vi "recorder.vi"() -> ()   [LabVIEW 2022 SP3]
uses:
  <vilib>/DAQmx/write.llb/DAQmx Write (Digital 1D Bool 1Chan 1Samp).vi
  <vilib>/Utility/file.llb/Write Delimited Spreadsheet (DBL).vi
  <vilib>/Utility/inputDevices.llb/keyboardAcquire.vi
  <vilib>/DAQmx/create/channels.llb/DAQmx Create Channel (DO-Digital Output).vi
  <vilib>/DAQmx/miscellaneous.llb/DAQmx Fill In Error Info.vi
panel:
  out "Array":dbl[](array[numeric])
  out "Numeric":dbl
  out "error out 97":errorcluster
  out "error out 96":errorcluster
  out "error out 95":errorcluster
  out "error out 94":errorcluster
  out "error out 93":errorcluster
  out "error out 92":errorcluster
  out "error out 91":errorcluster
  out "error out 90":errorcluster
  out "error out 89":errorcluster
  out "error out 88":errorcluster
  out "error out 87":errorcluster
  out "error out 86":errorcluster
  out "error out 85":errorcluster
  out "error out 84":errorcluster
  out "error out 83":errorcluster
  out "error out 82":errorcluster
  out "error out 81":errorcluster
  out "error out 80":errorcluster
  out "error out 79":errorcluster
  out "error out 78":errorcluster
  out "error out 77":errorcluster
  out "error out 76":errorcluster
  out "error out 75":errorcluster
  out "error out 74":errorcluster
  out "error out 73":errorcluster
  out "error out 72":errorcluster
  out "error out 71":errorcluster
  out "error out 70":errorcluster
  out "error out 69":errorcluster
  out "error out 68":errorcluster
  out "error out 67":errorcluster
  out "error out 66":errorcluster
  out "error out 65":errorcluster
  out "error out 64":errorcluster
  out "error out 63":errorcluster
  out "error out 62":errorcluster
  out "error out 61":errorcluster
  out "error out 60":errorcluster
  out "error out 59":errorcluster
  out "error out 58":errorcluster
  out "error out 57":errorcluster
  out "error out 56":errorcluster
  out "error out 55":errorcluster
  out "error out 54":errorcluster
  out "error out 53":errorcluster
  out "error out 52":errorcluster
  out "error out 51":errorcluster
  out "error out 50":errorcluster
  out "error out 49":errorcluster
  out "error out 48":errorcluster
  out "error out 47":errorcluster
  out "error out 46":errorcluster
  out "error out 45":errorcluster
  out "error out 44":errorcluster
  out "error out 43":errorcluster
  out "error out 42":errorcluster
  out "error out 41":errorcluster
  out "error out 40":errorcluster
  out "error out 39":errorcluster
  out "error out 38":errorcluster
  out "error out 37":errorcluster
  out "error out 36":errorcluster
  out "error out 35":errorcluster
  out "error out 34":errorcluster
  out "error out 33":errorcluster
  out "error out 32":errorcluster
  out "error out 31":errorcluster
  out "error out 30":errorcluster
  out "error out 29":errorcluster
  out "error out 28":errorcluster
  out "error out 27":errorcluster
  out "error out 26":errorcluster
  out "error out 18":errorcluster
  out "error out 19":errorcluster
  out "error out 20":errorcluster
  out "error out 21":errorcluster
  out "error out 22":errorcluster
  out "error out 23":errorcluster
  out "error out 24":errorcluster
  out "error out 25":errorcluster
  in  "stop":bool
  out "key":T1(ring)
  out "String":string
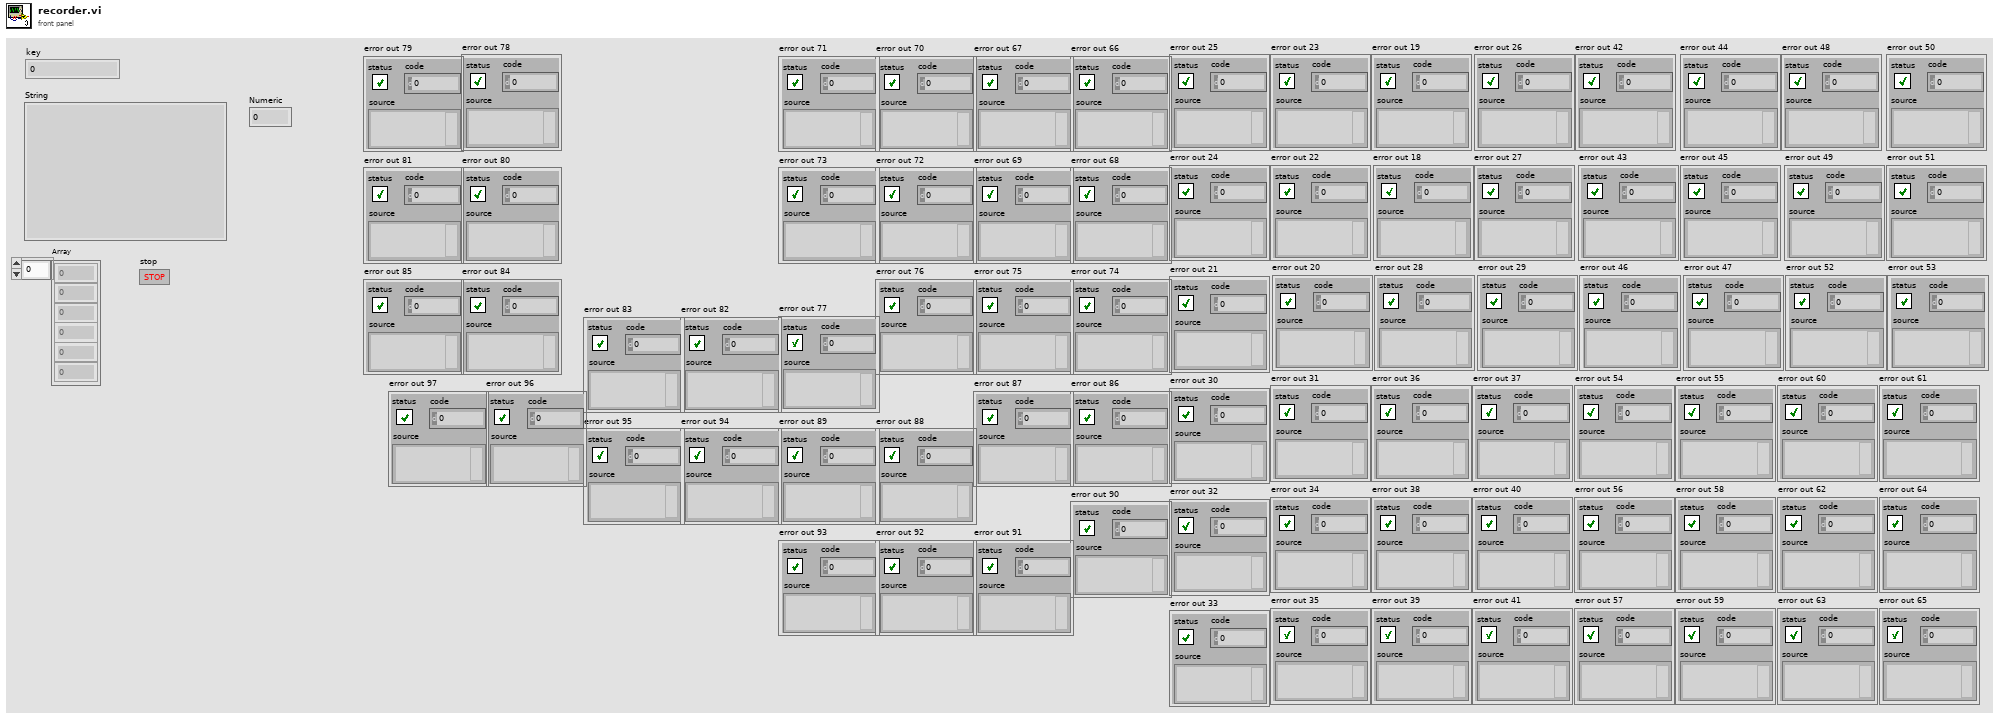
[diagram p1: front panel]
types:
  T1 = enum16{"0", "1", "2", "3", "4", "5", "6", "7", "8", "9", "A", "B", "C", "D", "E", "F", "G", "H", "I", "J", "K", "L", "M", "N", "O", "P", "Q", "R", "S", "T", "U", "V", "W", "X", "Y", "Z", "F1", "F2", "F3", "F4", "F5", "F6", "F7", "F8", "F9", "F10", "F11", "F12", "F13", "F14", "F15", "ADD", "BACK", "BACKSLASH", "CAPITAL", "COMMA", "DECIMAL", "DELETE", "DIVIDE", "DOWN", "END", "EQUALS", "ESCAPE", "GRAVE (`)", "HOME", "INSERT", "LBRACKET", "LCONTROL", "LEFT", "L ALT", "LSHIFT", "LWIN", "MINUS", "MULTIPLY", "NEXT", "NUMLOCK", "NUMPAD_0", "NUMPAD_1", "NUMPAD_2", "NUMPAD_3", "NUMPAD_4", "NUMPAD_5", "NUMPAD_6", "NUMPAD_7", "NUMPAD_8", "NUMPAD_9", "PAUSE", "PERIOD", "PRIOR (PG UP)", "RBRACKET", "RCONTROL", "RETURN", "RIGHT", "R ALT", "RSHIFT", "RWIN", "SCROLL", "SEMICOLON", "SLASH", "SPACE", "SUBTRACT", "TAB", "UP", "ENTER (num pad)", "' (quote)"}
  T2 = enum16{"0", "1", "2", "3", "4", "5", "6", "7", "8", "9", "A", "B", "C", "D", "E", "F", "G", "H", "I", "J", "K", "L", "M", "N", "O", "P", "Q", "R", "S", "T", "U", "V", "W", "X", "Y", "Z", "F1", "F2", "F3", "F4", "F5", "F6", "F7", "F8", "F9", "F10", "F11", "F12", "F13", "F14", "F15", "ADD", "BACK", "BACKSLASH", "CAPITAL", "COMMA", "DECIMAL", "DELETE", "DIVIDE", "DOWN", "END", "EQUALS", "ESCAPE", "GRAVE (`)", "HOME", "INSERT", "LBRACKET", "LCONTROL", "LEFT", "L ALT", "LSHIFT", "LWIN", "MINUS", "MULTIPLY", "NEXT", "NUMLOCK", "NUMPAD_0", "NUMPAD_1", "NUMPAD_2", "NUMPAD_3", "NUMPAD_4", "NUMPAD_5", "NUMPAD_6", "NUMPAD_7", "NUMPAD_8", "NUMPAD_9", "PAUSE", "PERIOD", "PRIOR (PG UP)", "RBRACKET", "RCONTROL", "RETURN", "RIGHT", "R ALT", "RSHIFT", "RWIN", "SCROLL", "SEMICOLON", "SLASH", "SPACE", "SUBTRACT", "TAB", "UP", "ENTER (num pad)", "' (quote)"}[]
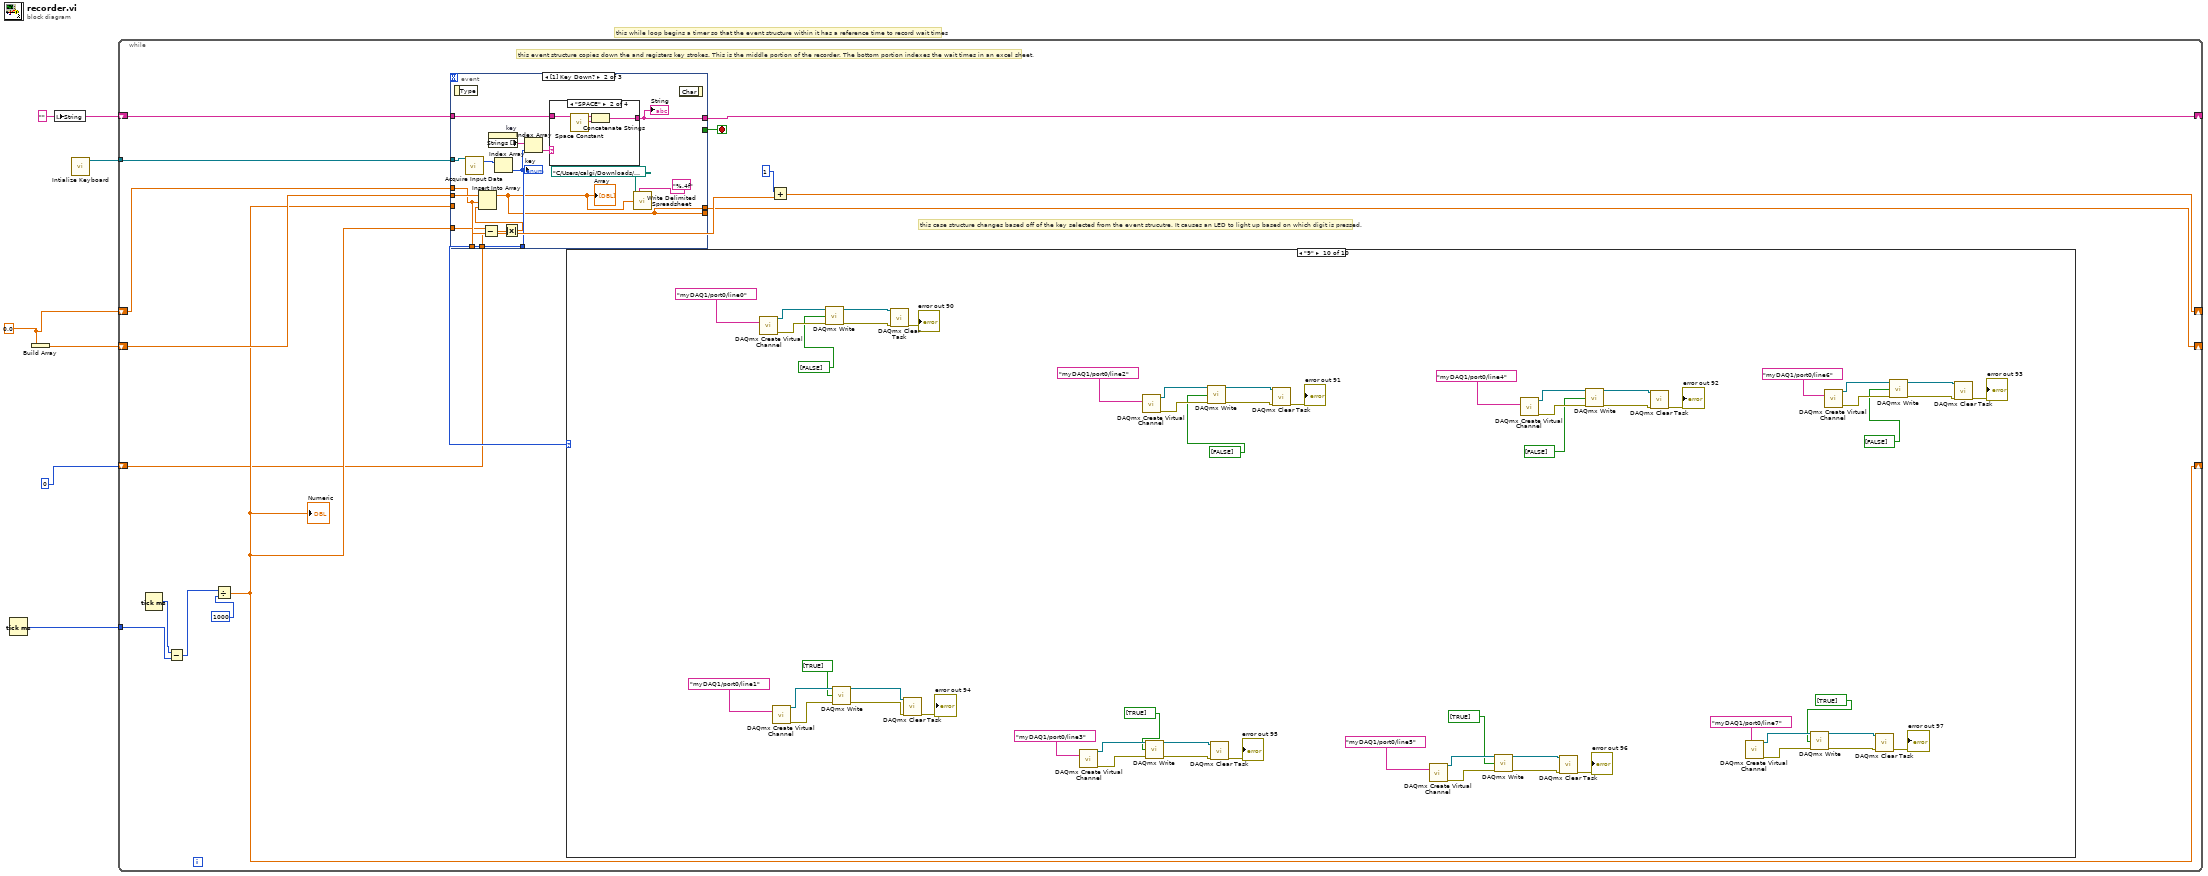
[diagram p0: block diagram]
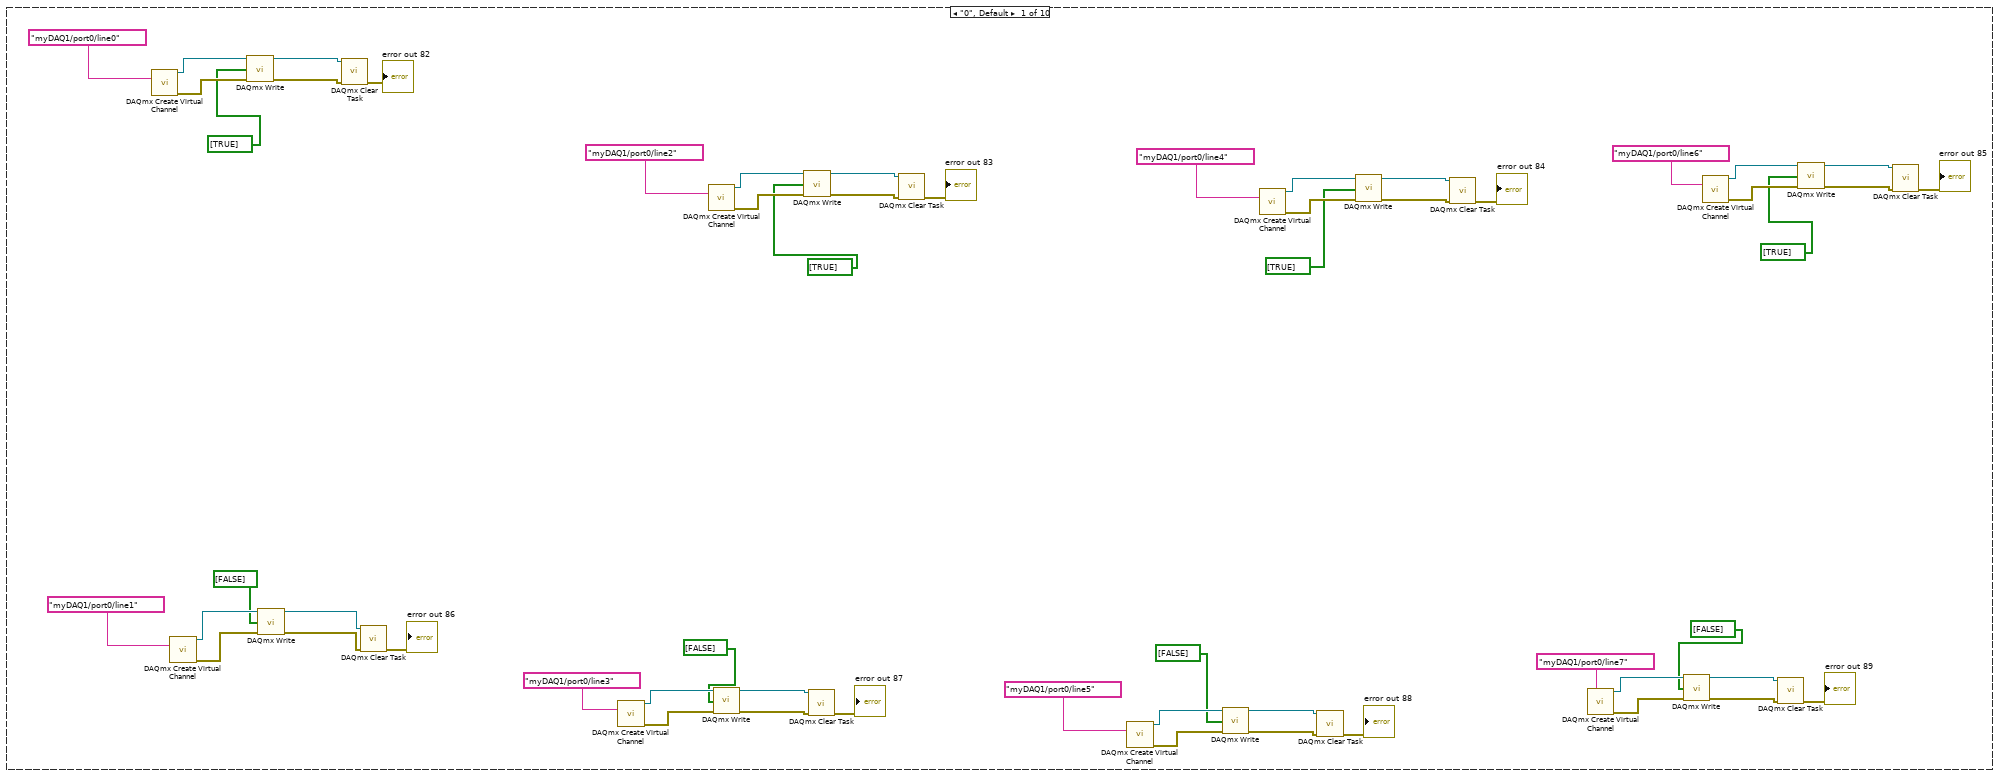
[diagram p2: hidden frame]
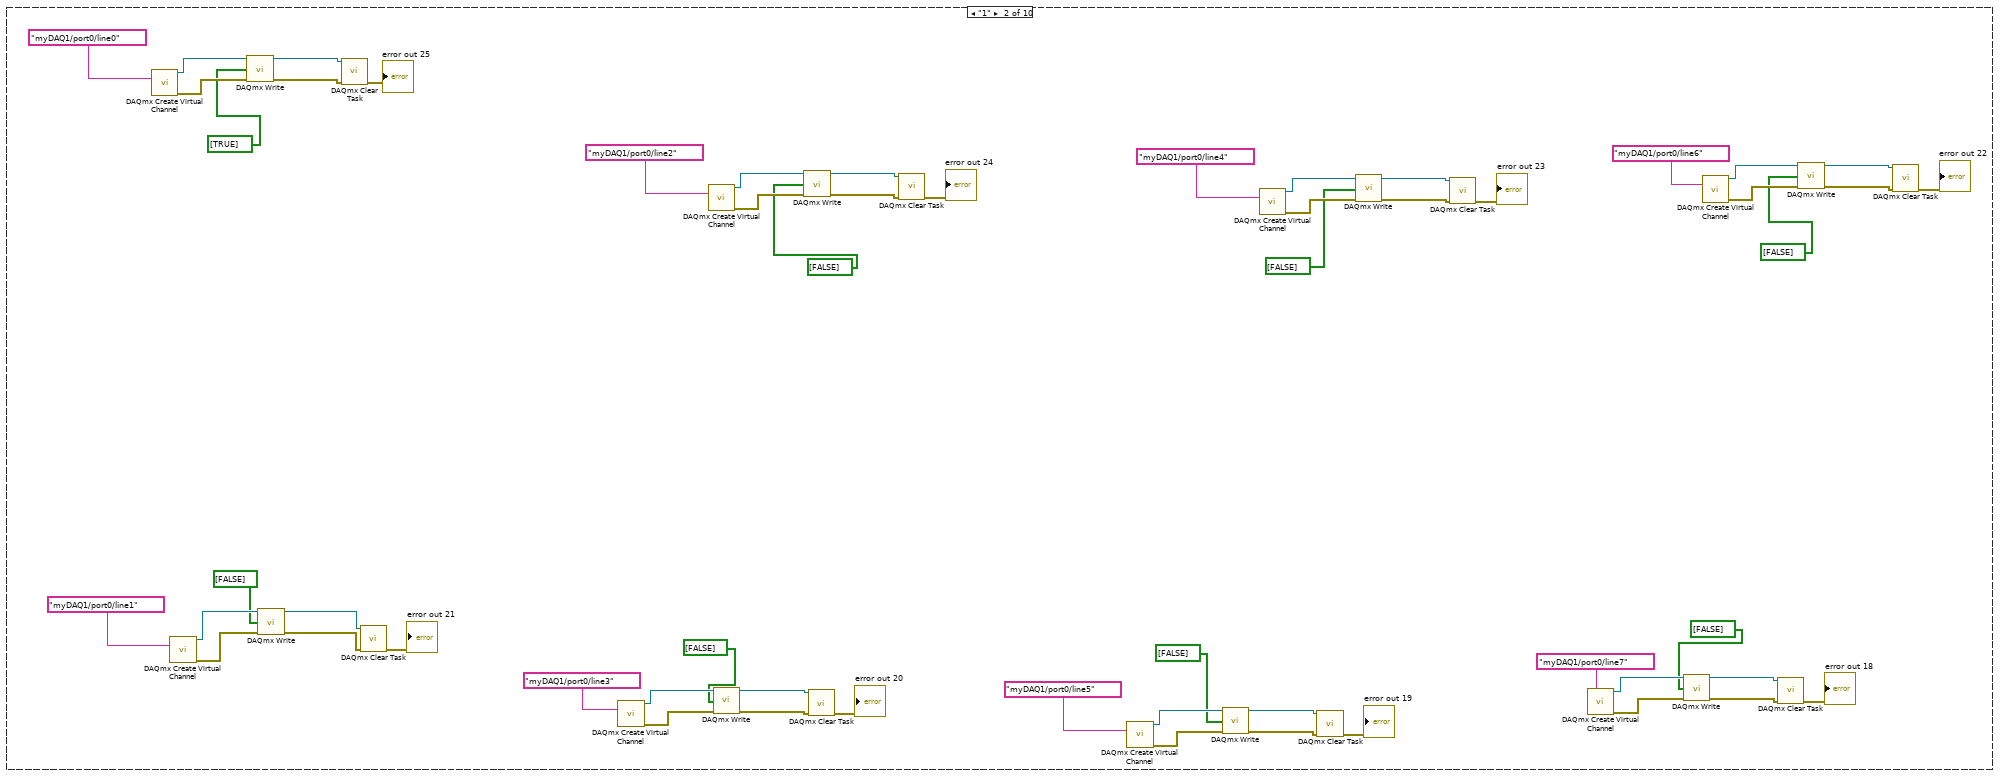
[diagram p3: hidden frame]
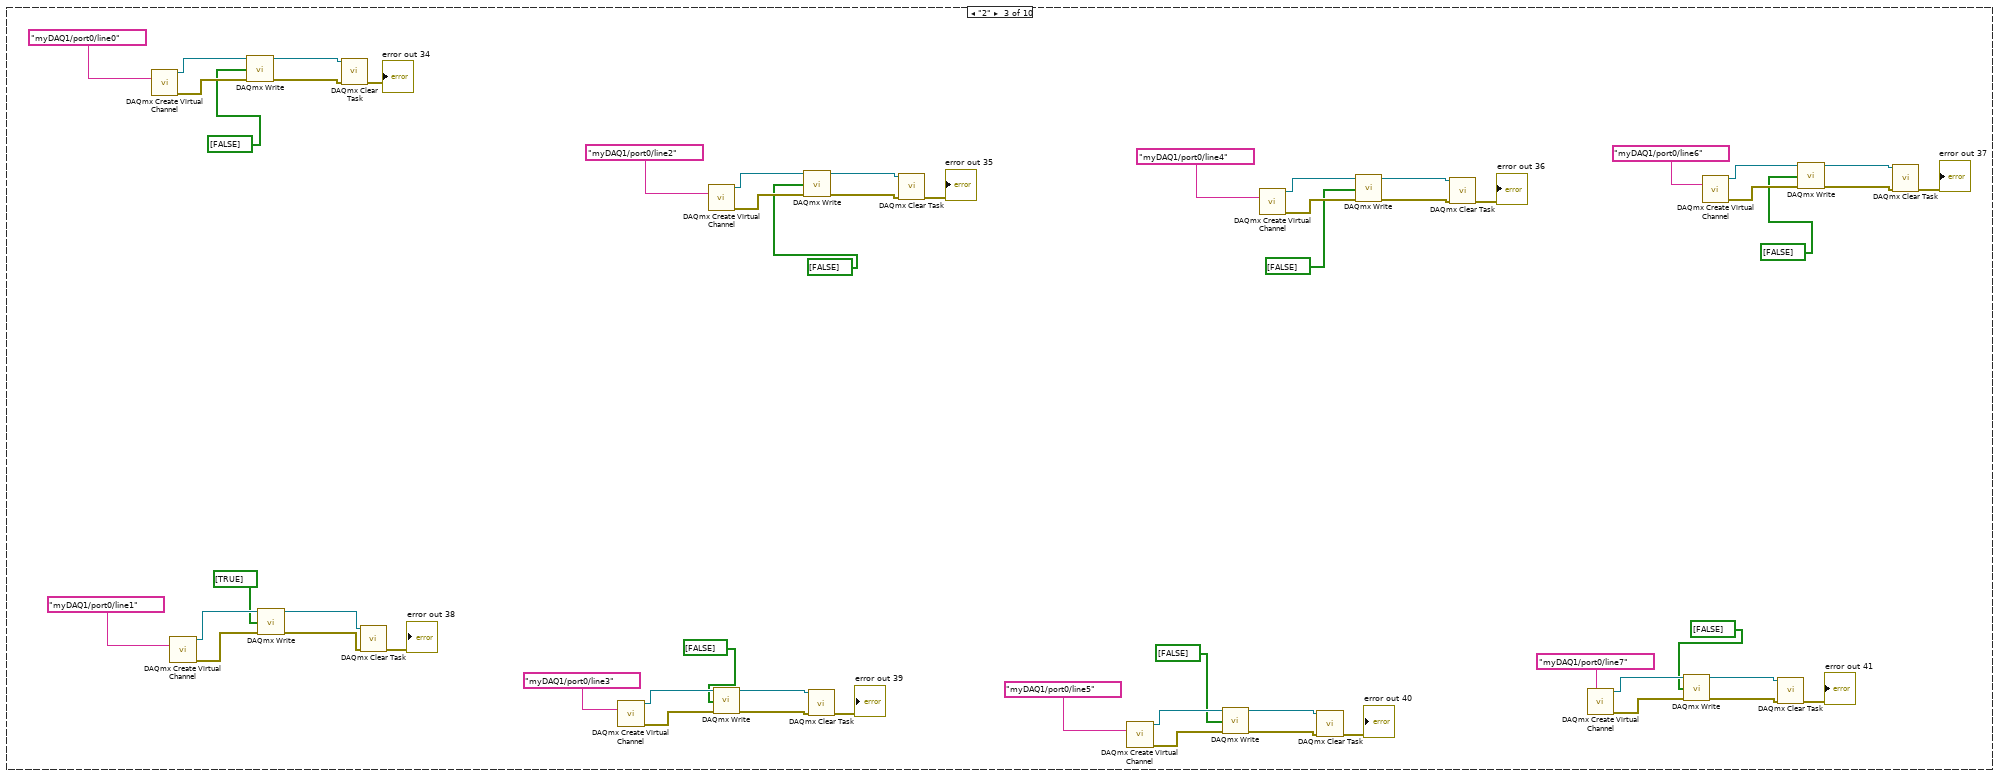
[diagram p4: hidden frame]
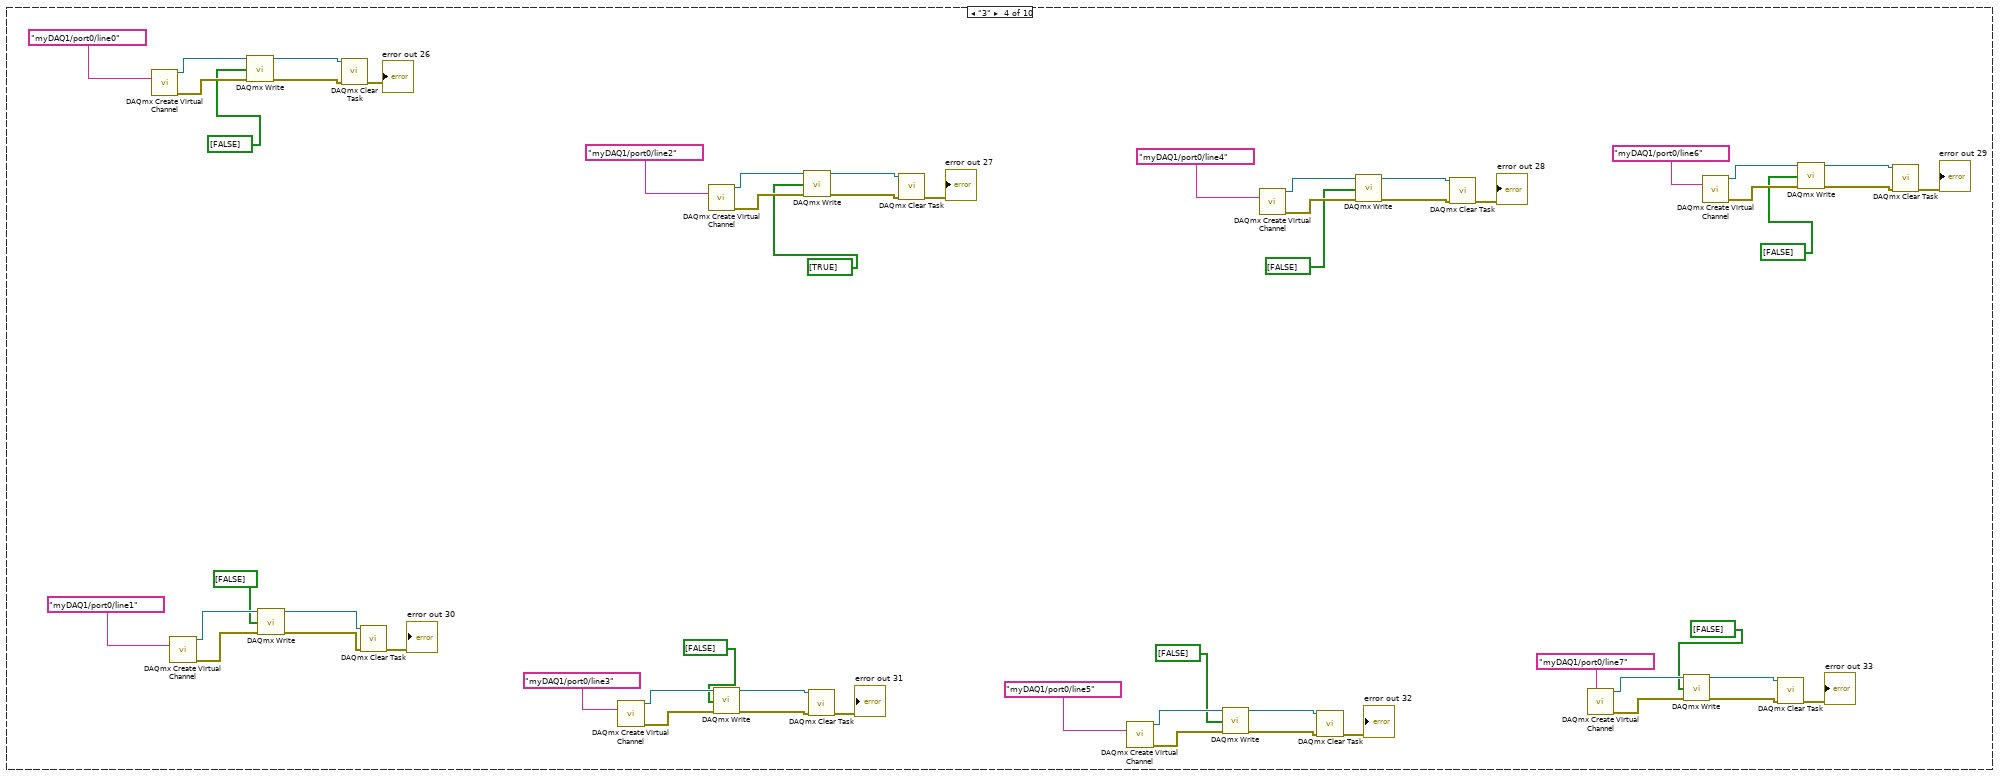
[diagram p5: hidden frame]
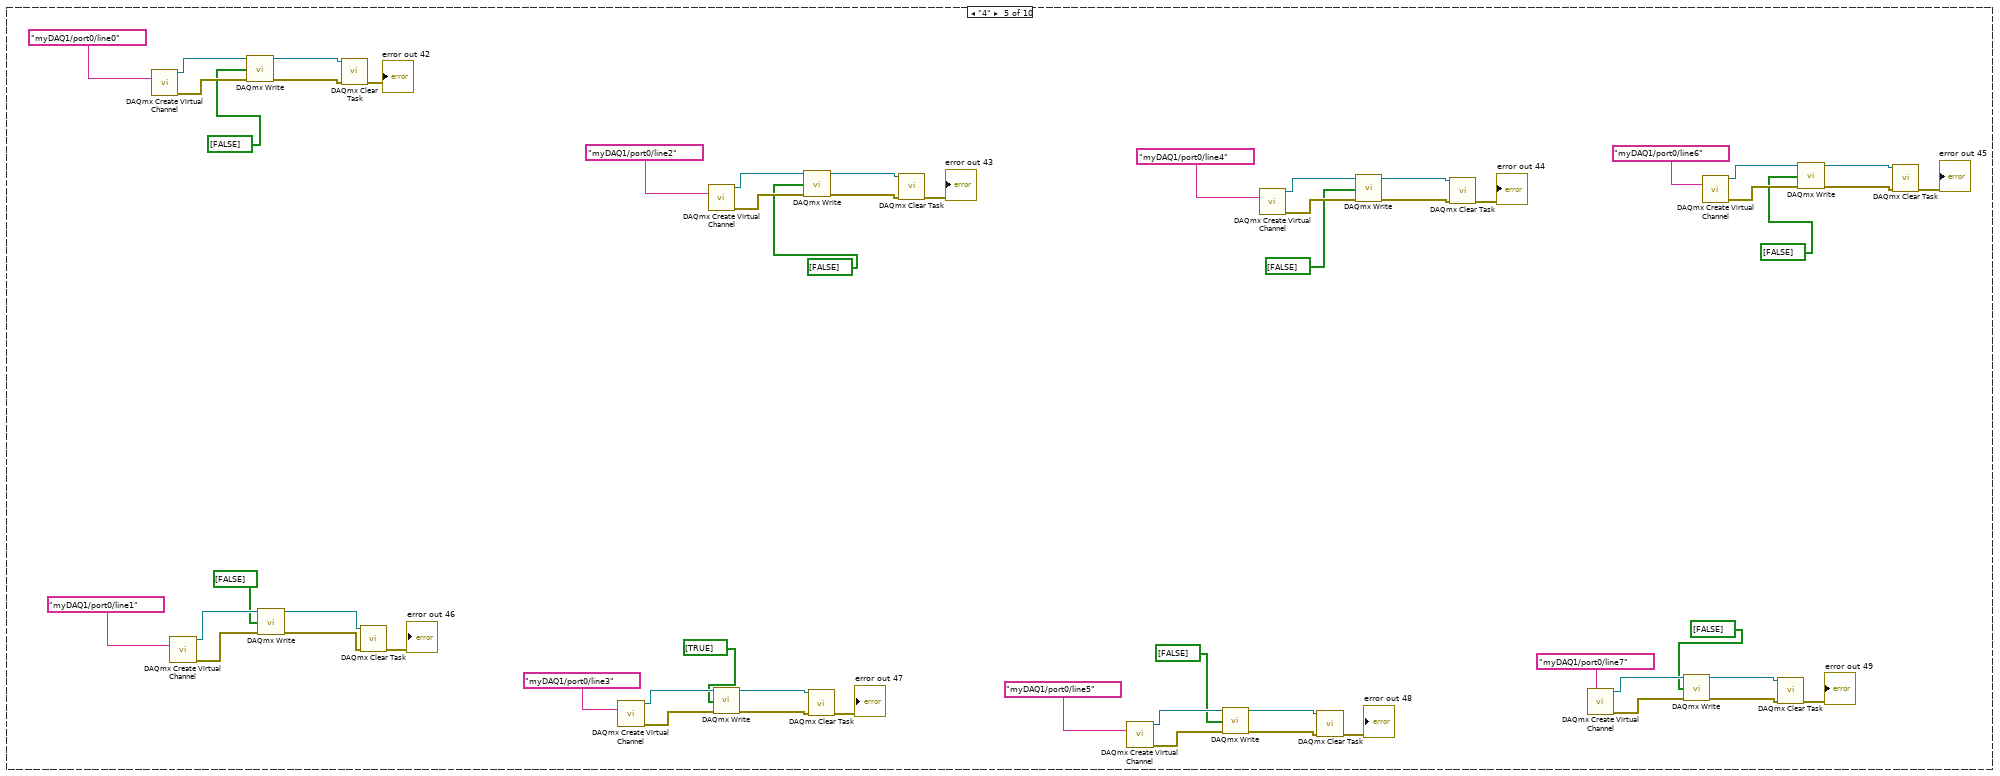
[diagram p6: hidden frame]
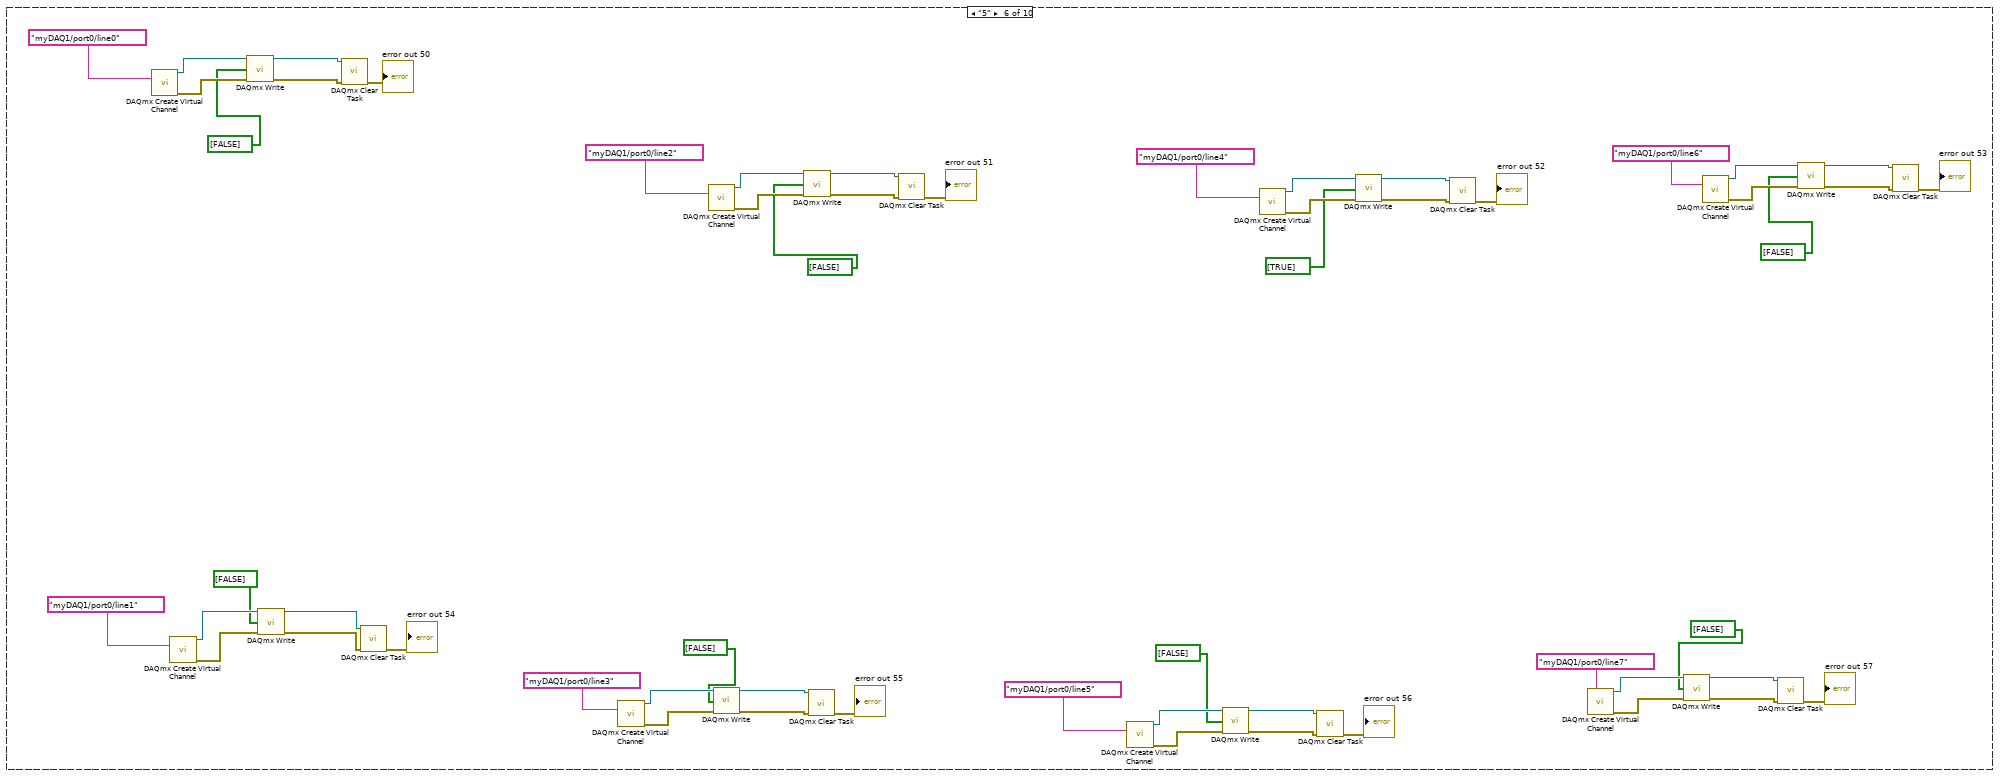
[diagram p7: hidden frame]
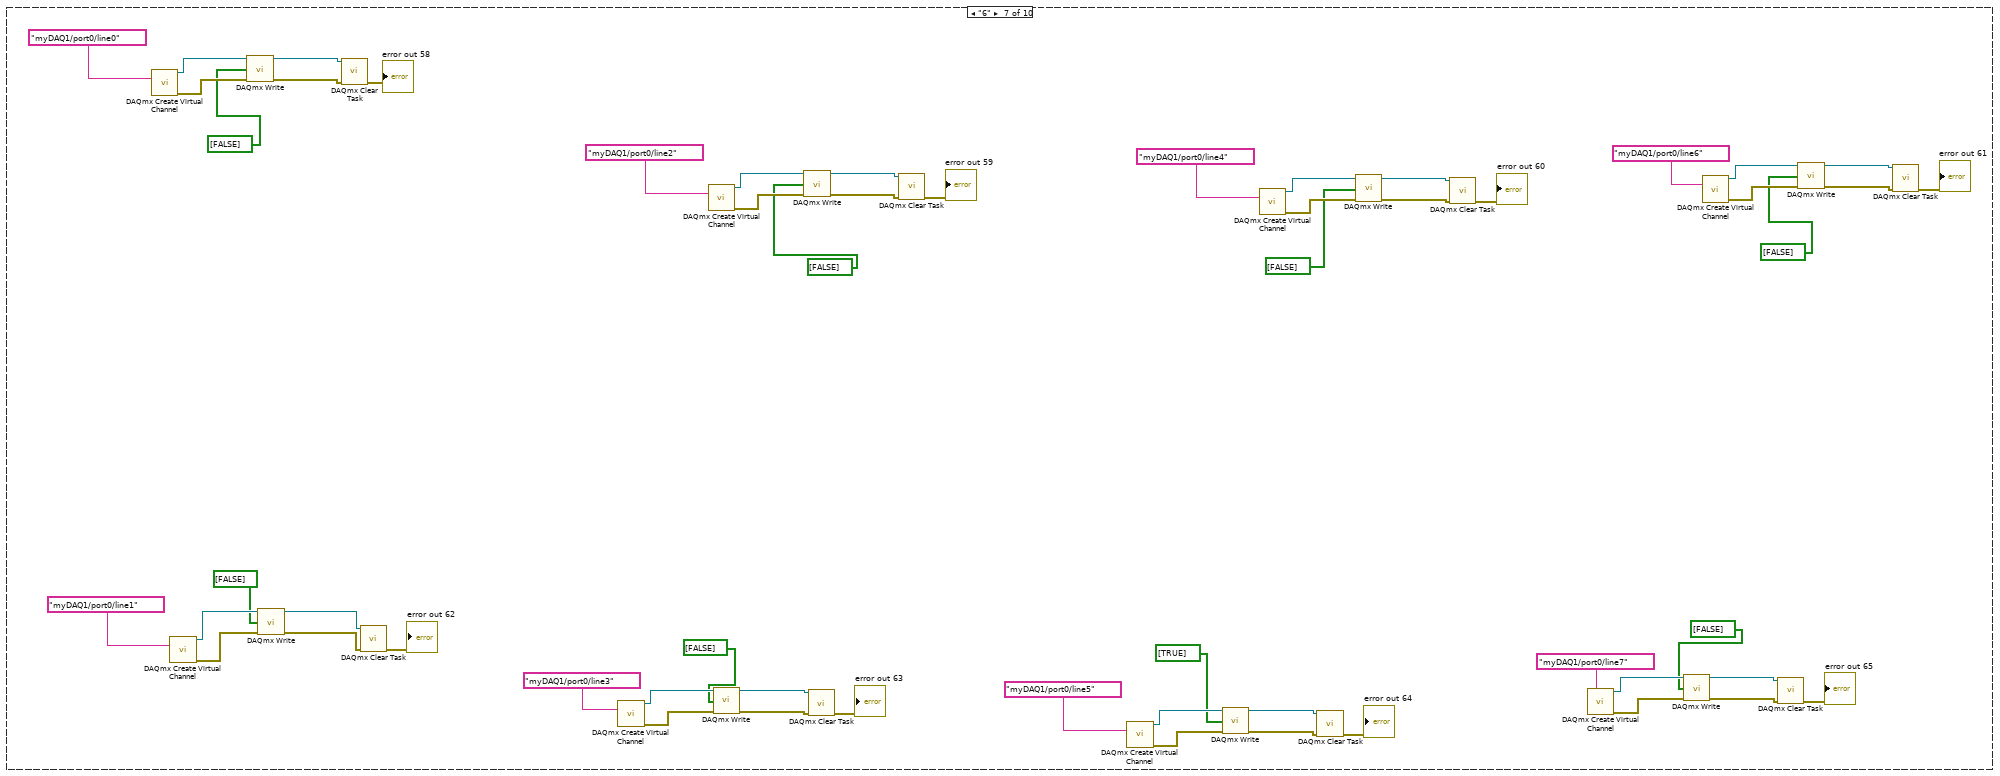
[diagram p8: hidden frame]
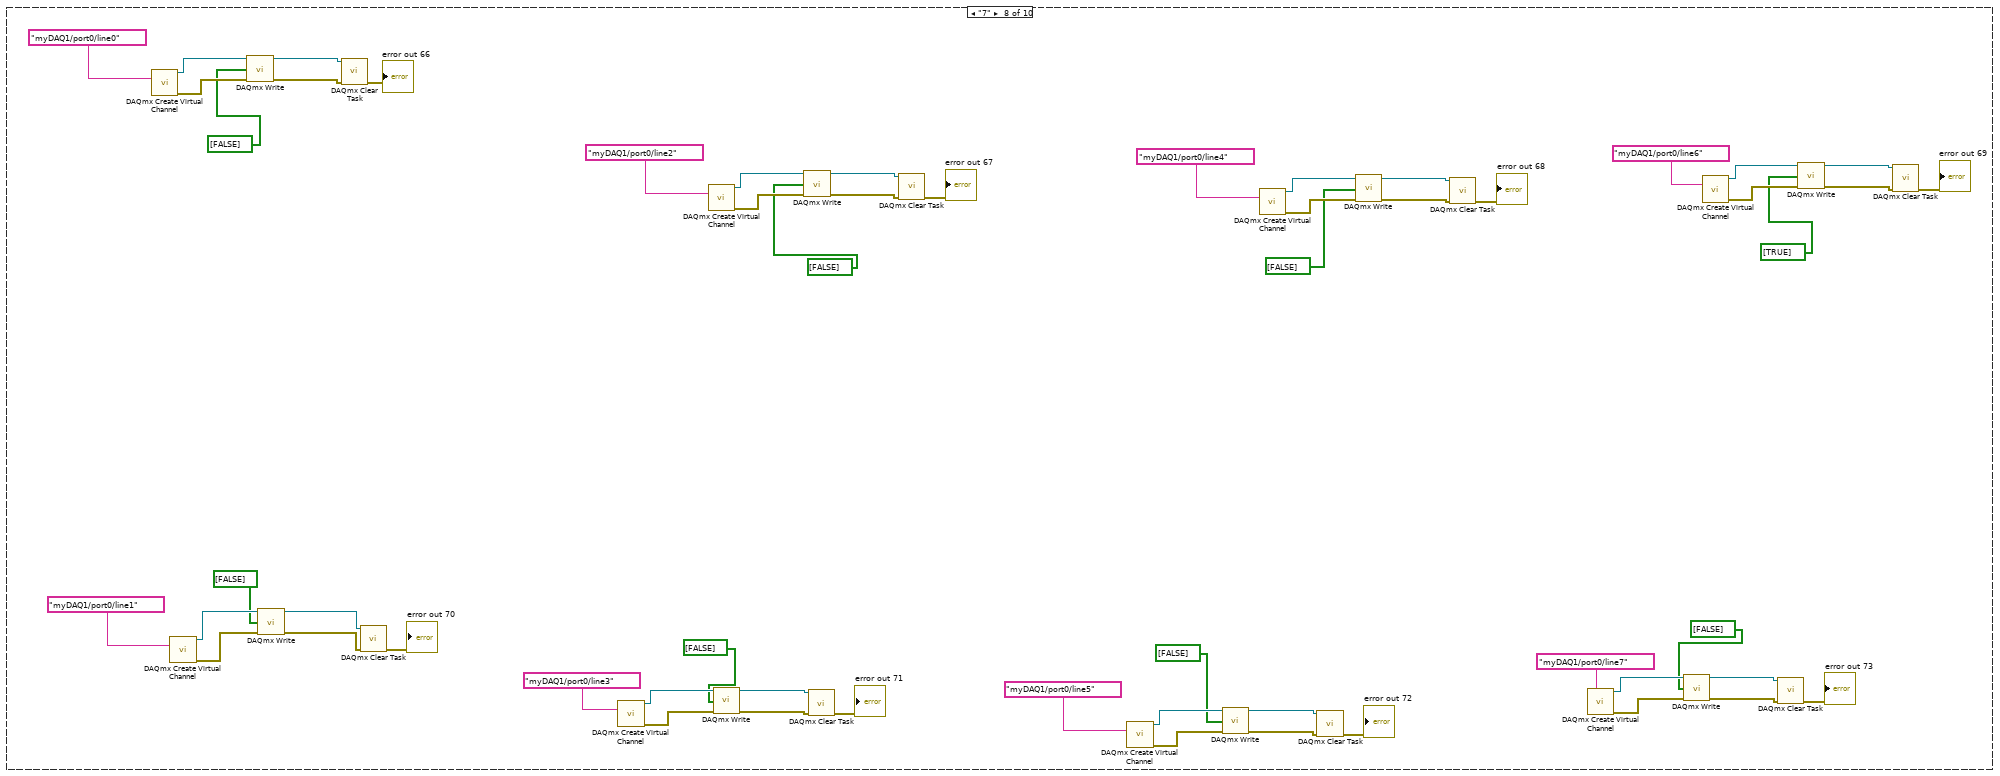
[diagram p9: hidden frame]
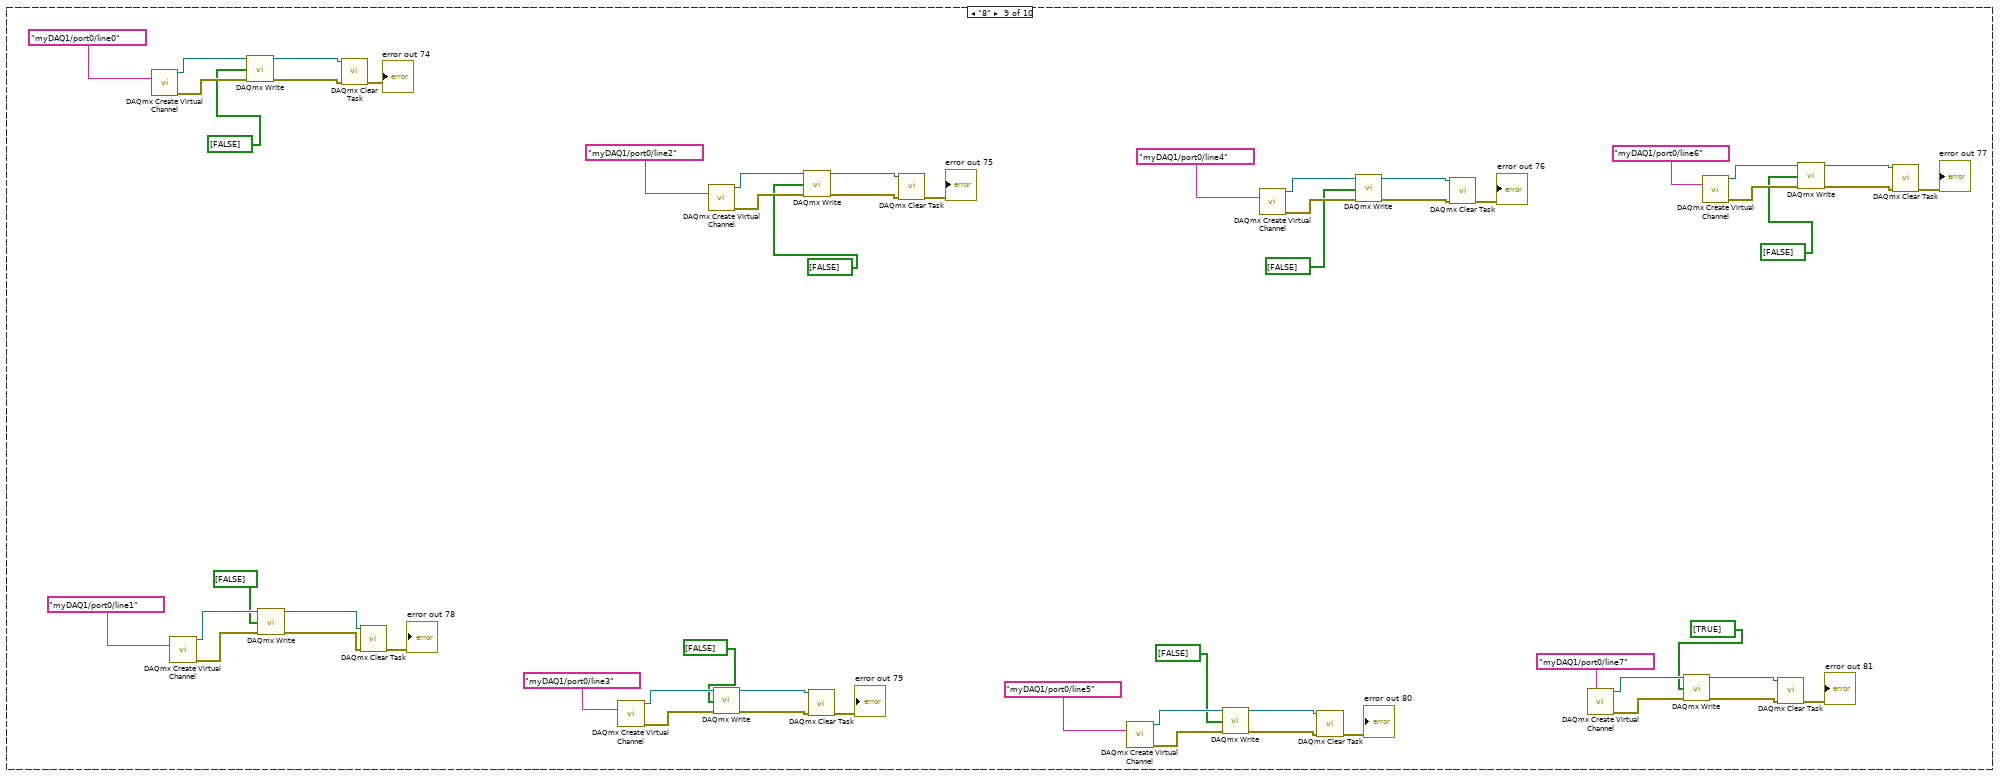
[diagram p10: hidden frame]
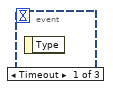
[diagram p11: hidden frame]
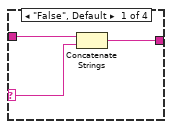
[diagram p12: hidden frame]
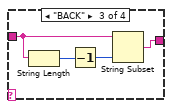
[diagram p13: hidden frame]
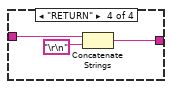
[diagram p14: hidden frame]
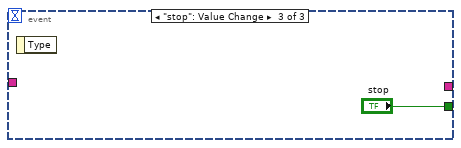
[diagram p15: hidden frame]
diagram:
  w2 = 0.0
  w5 = ""
  # "this while loop begins a timer so that the event structure within it has a reference time to record wait times"
  n1 = Tick Count (ms)() -> (millisecond timer value=w4:u32)
  n2 = Build Array(w2) -> (w3:dbl[])
  n3 = local write "String"(w5) -> ()
  n4 = call <vilib>:"Intialize Keyboard.vi"() -> ("device ID"=w6:refnum<k1>)  [unwired: 10 in, 1 out]
  n5 = while {
    tunnel: w6 -> [w22]
    shift-right: [w21] -> _
    shift-left: w5 -> [w20]
    tunnel: w4 -> [w18]
    shift-right: [w9] -> _
    shift-left: w3 -> [w14]
    shift-right: [w10] -> _
    shift-left: w2 -> [w12]
    shift-right: [w8] -> _
    shift-left: 0 -> [w7]
    stop <- w23 stop-if-true
    # "this case structure changes based off of the key selected from the event strucutre. It causes an LED to light up based on which digit is pressed."
    # "this event structure copies down the and registers key strokes. This is the middle portion of the recorder. The bottom portion indexes the wait times in an excel sheet."
    n6 = Tick Count (ms)() -> (millisecond timer value=w17:u32)
    n7 = Subtract(x=w17, y=w18) -> (x-y=w16:u32)
    n8 = Divide(x=w16, y=1000) -> (x/y=w8:dbl)
    "Numeric" <- w8
    n9 = event shown="[1] Key Down?" {
      selector: _ -> [_ _ _]
      dyn-events: _ -> [_ _ _]
      timeout: _ -> [_ _ _]
      tunnel: [_ _ "stop"] -> w23
      tunnel: w22 -> [_ w599 _]
      tunnel: [_ w594 _] -> w21
      tunnel: w20 -> [_ w595 _]
      tunnel: [_ w593 _] -> w19
      tunnel: w8 -> [_ _ _]
      tunnel: [_ w588 _] -> _
      tunnel: w14 -> [_ w590 _]
      tunnel: w12 -> [_ w589 _]
      tunnel: [_ w589 _] -> w11
      tunnel: [_ w588 _] -> w9
      tunnel: w8 -> [_ w587 _]
      tunnel: w7 -> [_ w586 _]
      event Timeout {
        n10 = event-data() -> ()  [unwired: 1 in, 1 out]
      }
      event Key Down? {
        n11 = event-data() -> ()  [unwired: 1 in, 1 out]
        n12 = call-poly <vilib>:"Acquire Input Data.vi"("device ID"=w599) -> ("keys pressed"=w598:T2)  [unwired: 16 in, 2 out]
        n13 = Subtract(x=w587, y=w586) -> (x-y=w585:dbl)
        n14 = property on="key" class="Enum (strict)"() -> ("Strings []"=w597:string[])  [unwired: 2 in, 2 out]
        n15 = Index Array(array=w598) -> (element=w593:T1)  [unwired: 1 in]
        "key" <- w593
        n16 = Absolute Value(x=w585) -> (abs(x)=w584:dbl)
        n17 = Insert Into Array(array=w590, index=w589, new element=w584) -> (w588:dbl[])
        "Array" <- w588
        n18 = Index Array(array=w597, index=w593) -> (element=w596:string)
        n19 = case shown="\"SPACE\"" w596 {
          selector: w596 -> [w600 _ _ _]
          tunnel: w595 -> [w602 w605 w609 w612]
          tunnel: [w601 w603 w607 w610] -> w594
          frame "False", Default {
            n20 = Concatenate Strings(w602, w600) -> (w601:string)
          }
          frame "SPACE" {
            n21 = call <vilib>:"Space Constant.vi"() -> ("String"=w604:string)
            n22 = Concatenate Strings(w605, w604) -> (w603:string)
          }
          frame "BACK" {
            n23 = String Length(string=w609) -> (length=w608:i32)
            n24 = Decrement(x=w608) -> (x-1=w606:i32)
            n25 = String Subset(string=w609, length (rest)=w606) -> (substring=w607:string)  [unwired: 1 in]
          }
          frame "RETURN" {
            n26 = Concatenate Strings(w612, "\r\n") -> (w610:string)
          }
        }
        "String" <- w594
        n27 = call-poly <vilib>:"Write Delimited Spreadsheet.vi"("file path (dialog if empty)"=path "C:/Users/calgi/Downloads/keyboardpatternBeta.csv", "format (%.3f)"="%.4f", "1D data"=w588) -> ()  [unwired: 11 in, 2 out]
        n28 = event-data() -> ()  [unwired: 2 in, 1 out]
      }
      event "stop": Value Change {
        n29 = event-data() -> ()  [unwired: 1 in, 1 out]
      }
    }
    n30 = case shown="\"9\"" w19 {
      frame "0", Default {
        n31 = call-poly <vilib>:"DAQmx Create Virtual Channel.vi"("lines"=tag "myDAQ1/port0/line0") -> ("task out"=w79:refnum<k21>, "error out"=w77:errorcluster)  [unwired: 13 in]
        n32 = call-poly <vilib>:"DAQmx Create Virtual Channel.vi"("lines"=tag "myDAQ1/port0/line1") -> ("task out"=w55:refnum<k21>, "error out"=w53:errorcluster)  [unwired: 13 in]
        n33 = call-poly <vilib>:"DAQmx Write.vi"("task/channels in"=w79, "data"=bool[] [TRUE], "error in"=w77) -> ("task out"=w78:refnum<k21>, "error out"=w76:errorcluster)  [unwired: 10 in, 1 out]
        n34 = call-poly <vilib>:"DAQmx Write.vi"("task/channels in"=w55, "data"=bool[] [FALSE], "error in"=w53) -> ("task out"=w54:refnum<k21>, "error out"=w52:errorcluster)  [unwired: 10 in, 1 out]
        n35 = call <vilib>:"DAQmx Clear Task.vi"("task in"=w78, "error in"=w76) -> ("error out"=→"error out 82":errorcluster)  [unwired: 13 in]
        n36 = call <vilib>:"DAQmx Clear Task.vi"("task in"=w54, "error in"=w52) -> ("error out"=→"error out 86":errorcluster)  [unwired: 13 in]
        n37 = call-poly <vilib>:"DAQmx Create Virtual Channel.vi"("lines"=tag "myDAQ1/port0/line3") -> ("task out"=w49:refnum<k21>, "error out"=w47:errorcluster)  [unwired: 13 in]
        n38 = call-poly <vilib>:"DAQmx Create Virtual Channel.vi"("lines"=tag "myDAQ1/port0/line2") -> ("task out"=w73:refnum<k21>, "error out"=w71:errorcluster)  [unwired: 13 in]
        n39 = call-poly <vilib>:"DAQmx Write.vi"("task/channels in"=w49, "data"=bool[] [FALSE], "error in"=w47) -> ("task out"=w48:refnum<k21>, "error out"=w46:errorcluster)  [unwired: 10 in, 1 out]
        n40 = call-poly <vilib>:"DAQmx Write.vi"("task/channels in"=w73, "data"=bool[] [TRUE], "error in"=w71) -> ("task out"=w72:refnum<k21>, "error out"=w70:errorcluster)  [unwired: 10 in, 1 out]
        n41 = call <vilib>:"DAQmx Clear Task.vi"("task in"=w48, "error in"=w46) -> ("error out"=→"error out 87":errorcluster)  [unwired: 13 in]
        n42 = call <vilib>:"DAQmx Clear Task.vi"("task in"=w72, "error in"=w70) -> ("error out"=→"error out 83":errorcluster)  [unwired: 13 in]
        n43 = call-poly <vilib>:"DAQmx Create Virtual Channel.vi"("lines"=tag "myDAQ1/port0/line5") -> ("task out"=w43:refnum<k21>, "error out"=w41:errorcluster)  [unwired: 13 in]
        n44 = call-poly <vilib>:"DAQmx Write.vi"("task/channels in"=w43, "data"=bool[] [FALSE], "error in"=w41) -> ("task out"=w42:refnum<k21>, "error out"=w40:errorcluster)  [unwired: 10 in, 1 out]
        n45 = call-poly <vilib>:"DAQmx Create Virtual Channel.vi"("lines"=tag "myDAQ1/port0/line4") -> ("task out"=w67:refnum<k21>, "error out"=w65:errorcluster)  [unwired: 13 in]
        n46 = call <vilib>:"DAQmx Clear Task.vi"("task in"=w42, "error in"=w40) -> ("error out"=→"error out 88":errorcluster)  [unwired: 13 in]
        n47 = call-poly <vilib>:"DAQmx Write.vi"("task/channels in"=w67, "data"=bool[] [TRUE], "error in"=w65) -> ("task out"=w66:refnum<k21>, "error out"=w64:errorcluster)  [unwired: 10 in, 1 out]
        n48 = call <vilib>:"DAQmx Clear Task.vi"("task in"=w66, "error in"=w64) -> ("error out"=→"error out 84":errorcluster)  [unwired: 13 in]
        n49 = call-poly <vilib>:"DAQmx Create Virtual Channel.vi"("lines"=tag "myDAQ1/port0/line7") -> ("task out"=w37:refnum<k21>, "error out"=w35:errorcluster)  [unwired: 13 in]
        n50 = call-poly <vilib>:"DAQmx Write.vi"("task/channels in"=w37, "data"=bool[] [FALSE], "error in"=w35) -> ("task out"=w36:refnum<k21>, "error out"=w34:errorcluster)  [unwired: 10 in, 1 out]
        n51 = call-poly <vilib>:"DAQmx Create Virtual Channel.vi"("lines"=tag "myDAQ1/port0/line6") -> ("task out"=w61:refnum<k21>, "error out"=w59:errorcluster)  [unwired: 13 in]
        n52 = call <vilib>:"DAQmx Clear Task.vi"("task in"=w36, "error in"=w34) -> ("error out"=→"error out 89":errorcluster)  [unwired: 13 in]
        n53 = call-poly <vilib>:"DAQmx Write.vi"("task/channels in"=w61, "data"=bool[] [TRUE], "error in"=w59) -> ("task out"=w60:refnum<k21>, "error out"=w58:errorcluster)  [unwired: 10 in, 1 out]
        n54 = call <vilib>:"DAQmx Clear Task.vi"("task in"=w60, "error in"=w58) -> ("error out"=→"error out 85":errorcluster)  [unwired: 13 in]
      }
      frame "1" {
        n55 = call-poly <vilib>:"DAQmx Create Virtual Channel.vi"("lines"=tag "myDAQ1/port0/line0") -> ("task out"=w135:refnum<k21>, "error out"=w133:errorcluster)  [unwired: 13 in]
        n56 = call-poly <vilib>:"DAQmx Create Virtual Channel.vi"("lines"=tag "myDAQ1/port0/line1") -> ("task out"=w111:refnum<k21>, "error out"=w109:errorcluster)  [unwired: 13 in]
        n57 = call-poly <vilib>:"DAQmx Write.vi"("task/channels in"=w135, "data"=bool[] [TRUE], "error in"=w133) -> ("task out"=w134:refnum<k21>, "error out"=w132:errorcluster)  [unwired: 10 in, 1 out]
        n58 = call-poly <vilib>:"DAQmx Write.vi"("task/channels in"=w111, "data"=bool[] [FALSE], "error in"=w109) -> ("task out"=w110:refnum<k21>, "error out"=w108:errorcluster)  [unwired: 10 in, 1 out]
        n59 = call <vilib>:"DAQmx Clear Task.vi"("task in"=w134, "error in"=w132) -> ("error out"=→"error out 25":errorcluster)  [unwired: 13 in]
        n60 = call <vilib>:"DAQmx Clear Task.vi"("task in"=w110, "error in"=w108) -> ("error out"=→"error out 21":errorcluster)  [unwired: 13 in]
        n61 = call-poly <vilib>:"DAQmx Create Virtual Channel.vi"("lines"=tag "myDAQ1/port0/line3") -> ("task out"=w105:refnum<k21>, "error out"=w103:errorcluster)  [unwired: 13 in]
        n62 = call-poly <vilib>:"DAQmx Create Virtual Channel.vi"("lines"=tag "myDAQ1/port0/line2") -> ("task out"=w129:refnum<k21>, "error out"=w127:errorcluster)  [unwired: 13 in]
        n63 = call-poly <vilib>:"DAQmx Write.vi"("task/channels in"=w105, "data"=bool[] [FALSE], "error in"=w103) -> ("task out"=w104:refnum<k21>, "error out"=w102:errorcluster)  [unwired: 10 in, 1 out]
        n64 = call-poly <vilib>:"DAQmx Write.vi"("task/channels in"=w129, "data"=bool[] [FALSE], "error in"=w127) -> ("task out"=w128:refnum<k21>, "error out"=w126:errorcluster)  [unwired: 10 in, 1 out]
        n65 = call <vilib>:"DAQmx Clear Task.vi"("task in"=w104, "error in"=w102) -> ("error out"=→"error out 20":errorcluster)  [unwired: 13 in]
        n66 = call <vilib>:"DAQmx Clear Task.vi"("task in"=w128, "error in"=w126) -> ("error out"=→"error out 24":errorcluster)  [unwired: 13 in]
        n67 = call-poly <vilib>:"DAQmx Create Virtual Channel.vi"("lines"=tag "myDAQ1/port0/line5") -> ("task out"=w99:refnum<k21>, "error out"=w97:errorcluster)  [unwired: 13 in]
        n68 = call-poly <vilib>:"DAQmx Write.vi"("task/channels in"=w99, "data"=bool[] [FALSE], "error in"=w97) -> ("task out"=w98:refnum<k21>, "error out"=w96:errorcluster)  [unwired: 10 in, 1 out]
        n69 = call-poly <vilib>:"DAQmx Create Virtual Channel.vi"("lines"=tag "myDAQ1/port0/line4") -> ("task out"=w123:refnum<k21>, "error out"=w121:errorcluster)  [unwired: 13 in]
        n70 = call <vilib>:"DAQmx Clear Task.vi"("task in"=w98, "error in"=w96) -> ("error out"=→"error out 19":errorcluster)  [unwired: 13 in]
        n71 = call-poly <vilib>:"DAQmx Write.vi"("task/channels in"=w123, "data"=bool[] [FALSE], "error in"=w121) -> ("task out"=w122:refnum<k21>, "error out"=w120:errorcluster)  [unwired: 10 in, 1 out]
        n72 = call <vilib>:"DAQmx Clear Task.vi"("task in"=w122, "error in"=w120) -> ("error out"=→"error out 23":errorcluster)  [unwired: 13 in]
        n73 = call-poly <vilib>:"DAQmx Create Virtual Channel.vi"("lines"=tag "myDAQ1/port0/line7") -> ("task out"=w93:refnum<k21>, "error out"=w91:errorcluster)  [unwired: 13 in]
        n74 = call-poly <vilib>:"DAQmx Write.vi"("task/channels in"=w93, "data"=bool[] [FALSE], "error in"=w91) -> ("task out"=w92:refnum<k21>, "error out"=w90:errorcluster)  [unwired: 10 in, 1 out]
        n75 = call-poly <vilib>:"DAQmx Create Virtual Channel.vi"("lines"=tag "myDAQ1/port0/line6") -> ("task out"=w117:refnum<k21>, "error out"=w115:errorcluster)  [unwired: 13 in]
        n76 = call <vilib>:"DAQmx Clear Task.vi"("task in"=w92, "error in"=w90) -> ("error out"=→"error out 18":errorcluster)  [unwired: 13 in]
        n77 = call-poly <vilib>:"DAQmx Write.vi"("task/channels in"=w117, "data"=bool[] [FALSE], "error in"=w115) -> ("task out"=w116:refnum<k21>, "error out"=w114:errorcluster)  [unwired: 10 in, 1 out]
        n78 = call <vilib>:"DAQmx Clear Task.vi"("task in"=w116, "error in"=w114) -> ("error out"=→"error out 22":errorcluster)  [unwired: 13 in]
      }
      frame "2" {
        n79 = call-poly <vilib>:"DAQmx Create Virtual Channel.vi"("lines"=tag "myDAQ1/port0/line0") -> ("task out"=w191:refnum<k21>, "error out"=w189:errorcluster)  [unwired: 13 in]
        n80 = call-poly <vilib>:"DAQmx Create Virtual Channel.vi"("lines"=tag "myDAQ1/port0/line1") -> ("task out"=w167:refnum<k21>, "error out"=w165:errorcluster)  [unwired: 13 in]
        n81 = call-poly <vilib>:"DAQmx Write.vi"("task/channels in"=w191, "data"=bool[] [FALSE], "error in"=w189) -> ("task out"=w190:refnum<k21>, "error out"=w188:errorcluster)  [unwired: 10 in, 1 out]
        n82 = call-poly <vilib>:"DAQmx Write.vi"("task/channels in"=w167, "data"=bool[] [TRUE], "error in"=w165) -> ("task out"=w166:refnum<k21>, "error out"=w164:errorcluster)  [unwired: 10 in, 1 out]
        n83 = call <vilib>:"DAQmx Clear Task.vi"("task in"=w190, "error in"=w188) -> ("error out"=→"error out 34":errorcluster)  [unwired: 13 in]
        n84 = call <vilib>:"DAQmx Clear Task.vi"("task in"=w166, "error in"=w164) -> ("error out"=→"error out 38":errorcluster)  [unwired: 13 in]
        n85 = call-poly <vilib>:"DAQmx Create Virtual Channel.vi"("lines"=tag "myDAQ1/port0/line3") -> ("task out"=w161:refnum<k21>, "error out"=w159:errorcluster)  [unwired: 13 in]
        n86 = call-poly <vilib>:"DAQmx Create Virtual Channel.vi"("lines"=tag "myDAQ1/port0/line2") -> ("task out"=w185:refnum<k21>, "error out"=w183:errorcluster)  [unwired: 13 in]
        n87 = call-poly <vilib>:"DAQmx Write.vi"("task/channels in"=w161, "data"=bool[] [FALSE], "error in"=w159) -> ("task out"=w160:refnum<k21>, "error out"=w158:errorcluster)  [unwired: 10 in, 1 out]
        n88 = call-poly <vilib>:"DAQmx Write.vi"("task/channels in"=w185, "data"=bool[] [FALSE], "error in"=w183) -> ("task out"=w184:refnum<k21>, "error out"=w182:errorcluster)  [unwired: 10 in, 1 out]
        n89 = call <vilib>:"DAQmx Clear Task.vi"("task in"=w160, "error in"=w158) -> ("error out"=→"error out 39":errorcluster)  [unwired: 13 in]
        n90 = call <vilib>:"DAQmx Clear Task.vi"("task in"=w184, "error in"=w182) -> ("error out"=→"error out 35":errorcluster)  [unwired: 13 in]
        n91 = call-poly <vilib>:"DAQmx Create Virtual Channel.vi"("lines"=tag "myDAQ1/port0/line5") -> ("task out"=w155:refnum<k21>, "error out"=w153:errorcluster)  [unwired: 13 in]
        n92 = call-poly <vilib>:"DAQmx Write.vi"("task/channels in"=w155, "data"=bool[] [FALSE], "error in"=w153) -> ("task out"=w154:refnum<k21>, "error out"=w152:errorcluster)  [unwired: 10 in, 1 out]
        n93 = call-poly <vilib>:"DAQmx Create Virtual Channel.vi"("lines"=tag "myDAQ1/port0/line4") -> ("task out"=w179:refnum<k21>, "error out"=w177:errorcluster)  [unwired: 13 in]
        n94 = call <vilib>:"DAQmx Clear Task.vi"("task in"=w154, "error in"=w152) -> ("error out"=→"error out 40":errorcluster)  [unwired: 13 in]
        n95 = call-poly <vilib>:"DAQmx Write.vi"("task/channels in"=w179, "data"=bool[] [FALSE], "error in"=w177) -> ("task out"=w178:refnum<k21>, "error out"=w176:errorcluster)  [unwired: 10 in, 1 out]
        n96 = call <vilib>:"DAQmx Clear Task.vi"("task in"=w178, "error in"=w176) -> ("error out"=→"error out 36":errorcluster)  [unwired: 13 in]
        n97 = call-poly <vilib>:"DAQmx Create Virtual Channel.vi"("lines"=tag "myDAQ1/port0/line7") -> ("task out"=w149:refnum<k21>, "error out"=w147:errorcluster)  [unwired: 13 in]
        n98 = call-poly <vilib>:"DAQmx Write.vi"("task/channels in"=w149, "data"=bool[] [FALSE], "error in"=w147) -> ("task out"=w148:refnum<k21>, "error out"=w146:errorcluster)  [unwired: 10 in, 1 out]
        n99 = call-poly <vilib>:"DAQmx Create Virtual Channel.vi"("lines"=tag "myDAQ1/port0/line6") -> ("task out"=w173:refnum<k21>, "error out"=w171:errorcluster)  [unwired: 13 in]
        n100 = call <vilib>:"DAQmx Clear Task.vi"("task in"=w148, "error in"=w146) -> ("error out"=→"error out 41":errorcluster)  [unwired: 13 in]
        n101 = call-poly <vilib>:"DAQmx Write.vi"("task/channels in"=w173, "data"=bool[] [FALSE], "error in"=w171) -> ("task out"=w172:refnum<k21>, "error out"=w170:errorcluster)  [unwired: 10 in, 1 out]
        n102 = call <vilib>:"DAQmx Clear Task.vi"("task in"=w172, "error in"=w170) -> ("error out"=→"error out 37":errorcluster)  [unwired: 13 in]
      }
      frame "3" {
        n103 = call-poly <vilib>:"DAQmx Create Virtual Channel.vi"("lines"=tag "myDAQ1/port0/line0") -> ("task out"=w247:refnum<k21>, "error out"=w245:errorcluster)  [unwired: 13 in]
        n104 = call-poly <vilib>:"DAQmx Create Virtual Channel.vi"("lines"=tag "myDAQ1/port0/line1") -> ("task out"=w223:refnum<k21>, "error out"=w221:errorcluster)  [unwired: 13 in]
        n105 = call-poly <vilib>:"DAQmx Write.vi"("task/channels in"=w247, "data"=bool[] [FALSE], "error in"=w245) -> ("task out"=w246:refnum<k21>, "error out"=w244:errorcluster)  [unwired: 10 in, 1 out]
        n106 = call-poly <vilib>:"DAQmx Write.vi"("task/channels in"=w223, "data"=bool[] [FALSE], "error in"=w221) -> ("task out"=w222:refnum<k21>, "error out"=w220:errorcluster)  [unwired: 10 in, 1 out]
        n107 = call <vilib>:"DAQmx Clear Task.vi"("task in"=w246, "error in"=w244) -> ("error out"=→"error out 26":errorcluster)  [unwired: 13 in]
        n108 = call <vilib>:"DAQmx Clear Task.vi"("task in"=w222, "error in"=w220) -> ("error out"=→"error out 30":errorcluster)  [unwired: 13 in]
        n109 = call-poly <vilib>:"DAQmx Create Virtual Channel.vi"("lines"=tag "myDAQ1/port0/line3") -> ("task out"=w217:refnum<k21>, "error out"=w215:errorcluster)  [unwired: 13 in]
        n110 = call-poly <vilib>:"DAQmx Create Virtual Channel.vi"("lines"=tag "myDAQ1/port0/line2") -> ("task out"=w241:refnum<k21>, "error out"=w239:errorcluster)  [unwired: 13 in]
        n111 = call-poly <vilib>:"DAQmx Write.vi"("task/channels in"=w217, "data"=bool[] [FALSE], "error in"=w215) -> ("task out"=w216:refnum<k21>, "error out"=w214:errorcluster)  [unwired: 10 in, 1 out]
        n112 = call-poly <vilib>:"DAQmx Write.vi"("task/channels in"=w241, "data"=bool[] [TRUE], "error in"=w239) -> ("task out"=w240:refnum<k21>, "error out"=w238:errorcluster)  [unwired: 10 in, 1 out]
        n113 = call <vilib>:"DAQmx Clear Task.vi"("task in"=w216, "error in"=w214) -> ("error out"=→"error out 31":errorcluster)  [unwired: 13 in]
        n114 = call <vilib>:"DAQmx Clear Task.vi"("task in"=w240, "error in"=w238) -> ("error out"=→"error out 27":errorcluster)  [unwired: 13 in]
        n115 = call-poly <vilib>:"DAQmx Create Virtual Channel.vi"("lines"=tag "myDAQ1/port0/line5") -> ("task out"=w211:refnum<k21>, "error out"=w209:errorcluster)  [unwired: 13 in]
        n116 = call-poly <vilib>:"DAQmx Write.vi"("task/channels in"=w211, "data"=bool[] [FALSE], "error in"=w209) -> ("task out"=w210:refnum<k21>, "error out"=w208:errorcluster)  [unwired: 10 in, 1 out]
        n117 = call-poly <vilib>:"DAQmx Create Virtual Channel.vi"("lines"=tag "myDAQ1/port0/line4") -> ("task out"=w235:refnum<k21>, "error out"=w233:errorcluster)  [unwired: 13 in]
        n118 = call <vilib>:"DAQmx Clear Task.vi"("task in"=w210, "error in"=w208) -> ("error out"=→"error out 32":errorcluster)  [unwired: 13 in]
        n119 = call-poly <vilib>:"DAQmx Write.vi"("task/channels in"=w235, "data"=bool[] [FALSE], "error in"=w233) -> ("task out"=w234:refnum<k21>, "error out"=w232:errorcluster)  [unwired: 10 in, 1 out]
        n120 = call <vilib>:"DAQmx Clear Task.vi"("task in"=w234, "error in"=w232) -> ("error out"=→"error out 28":errorcluster)  [unwired: 13 in]
        n121 = call-poly <vilib>:"DAQmx Create Virtual Channel.vi"("lines"=tag "myDAQ1/port0/line7") -> ("task out"=w205:refnum<k21>, "error out"=w203:errorcluster)  [unwired: 13 in]
        n122 = call-poly <vilib>:"DAQmx Write.vi"("task/channels in"=w205, "data"=bool[] [FALSE], "error in"=w203) -> ("task out"=w204:refnum<k21>, "error out"=w202:errorcluster)  [unwired: 10 in, 1 out]
        n123 = call-poly <vilib>:"DAQmx Create Virtual Channel.vi"("lines"=tag "myDAQ1/port0/line6") -> ("task out"=w229:refnum<k21>, "error out"=w227:errorcluster)  [unwired: 13 in]
        n124 = call <vilib>:"DAQmx Clear Task.vi"("task in"=w204, "error in"=w202) -> ("error out"=→"error out 33":errorcluster)  [unwired: 13 in]
        n125 = call-poly <vilib>:"DAQmx Write.vi"("task/channels in"=w229, "data"=bool[] [FALSE], "error in"=w227) -> ("task out"=w228:refnum<k21>, "error out"=w226:errorcluster)  [unwired: 10 in, 1 out]
        n126 = call <vilib>:"DAQmx Clear Task.vi"("task in"=w228, "error in"=w226) -> ("error out"=→"error out 29":errorcluster)  [unwired: 13 in]
      }
      frame "4" {
        n127 = call-poly <vilib>:"DAQmx Create Virtual Channel.vi"("lines"=tag "myDAQ1/port0/line0") -> ("task out"=w303:refnum<k21>, "error out"=w301:errorcluster)  [unwired: 13 in]
        n128 = call-poly <vilib>:"DAQmx Create Virtual Channel.vi"("lines"=tag "myDAQ1/port0/line1") -> ("task out"=w279:refnum<k21>, "error out"=w277:errorcluster)  [unwired: 13 in]
        n129 = call-poly <vilib>:"DAQmx Write.vi"("task/channels in"=w303, "data"=bool[] [FALSE], "error in"=w301) -> ("task out"=w302:refnum<k21>, "error out"=w300:errorcluster)  [unwired: 10 in, 1 out]
        n130 = call-poly <vilib>:"DAQmx Write.vi"("task/channels in"=w279, "data"=bool[] [FALSE], "error in"=w277) -> ("task out"=w278:refnum<k21>, "error out"=w276:errorcluster)  [unwired: 10 in, 1 out]
        n131 = call <vilib>:"DAQmx Clear Task.vi"("task in"=w302, "error in"=w300) -> ("error out"=→"error out 42":errorcluster)  [unwired: 13 in]
        n132 = call <vilib>:"DAQmx Clear Task.vi"("task in"=w278, "error in"=w276) -> ("error out"=→"error out 46":errorcluster)  [unwired: 13 in]
        n133 = call-poly <vilib>:"DAQmx Create Virtual Channel.vi"("lines"=tag "myDAQ1/port0/line3") -> ("task out"=w273:refnum<k21>, "error out"=w271:errorcluster)  [unwired: 13 in]
        n134 = call-poly <vilib>:"DAQmx Create Virtual Channel.vi"("lines"=tag "myDAQ1/port0/line2") -> ("task out"=w297:refnum<k21>, "error out"=w295:errorcluster)  [unwired: 13 in]
        n135 = call-poly <vilib>:"DAQmx Write.vi"("task/channels in"=w273, "data"=bool[] [TRUE], "error in"=w271) -> ("task out"=w272:refnum<k21>, "error out"=w270:errorcluster)  [unwired: 10 in, 1 out]
        n136 = call-poly <vilib>:"DAQmx Write.vi"("task/channels in"=w297, "data"=bool[] [FALSE], "error in"=w295) -> ("task out"=w296:refnum<k21>, "error out"=w294:errorcluster)  [unwired: 10 in, 1 out]
        n137 = call <vilib>:"DAQmx Clear Task.vi"("task in"=w272, "error in"=w270) -> ("error out"=→"error out 47":errorcluster)  [unwired: 13 in]
        n138 = call <vilib>:"DAQmx Clear Task.vi"("task in"=w296, "error in"=w294) -> ("error out"=→"error out 43":errorcluster)  [unwired: 13 in]
        n139 = call-poly <vilib>:"DAQmx Create Virtual Channel.vi"("lines"=tag "myDAQ1/port0/line5") -> ("task out"=w267:refnum<k21>, "error out"=w265:errorcluster)  [unwired: 13 in]
        n140 = call-poly <vilib>:"DAQmx Write.vi"("task/channels in"=w267, "data"=bool[] [FALSE], "error in"=w265) -> ("task out"=w266:refnum<k21>, "error out"=w264:errorcluster)  [unwired: 10 in, 1 out]
        n141 = call-poly <vilib>:"DAQmx Create Virtual Channel.vi"("lines"=tag "myDAQ1/port0/line4") -> ("task out"=w291:refnum<k21>, "error out"=w289:errorcluster)  [unwired: 13 in]
        n142 = call <vilib>:"DAQmx Clear Task.vi"("task in"=w266, "error in"=w264) -> ("error out"=→"error out 48":errorcluster)  [unwired: 13 in]
        n143 = call-poly <vilib>:"DAQmx Write.vi"("task/channels in"=w291, "data"=bool[] [FALSE], "error in"=w289) -> ("task out"=w290:refnum<k21>, "error out"=w288:errorcluster)  [unwired: 10 in, 1 out]
        n144 = call <vilib>:"DAQmx Clear Task.vi"("task in"=w290, "error in"=w288) -> ("error out"=→"error out 44":errorcluster)  [unwired: 13 in]
        n145 = call-poly <vilib>:"DAQmx Create Virtual Channel.vi"("lines"=tag "myDAQ1/port0/line7") -> ("task out"=w261:refnum<k21>, "error out"=w259:errorcluster)  [unwired: 13 in]
        n146 = call-poly <vilib>:"DAQmx Write.vi"("task/channels in"=w261, "data"=bool[] [FALSE], "error in"=w259) -> ("task out"=w260:refnum<k21>, "error out"=w258:errorcluster)  [unwired: 10 in, 1 out]
        n147 = call-poly <vilib>:"DAQmx Create Virtual Channel.vi"("lines"=tag "myDAQ1/port0/line6") -> ("task out"=w285:refnum<k21>, "error out"=w283:errorcluster)  [unwired: 13 in]
        n148 = call <vilib>:"DAQmx Clear Task.vi"("task in"=w260, "error in"=w258) -> ("error out"=→"error out 49":errorcluster)  [unwired: 13 in]
        n149 = call-poly <vilib>:"DAQmx Write.vi"("task/channels in"=w285, "data"=bool[] [FALSE], "error in"=w283) -> ("task out"=w284:refnum<k21>, "error out"=w282:errorcluster)  [unwired: 10 in, 1 out]
        n150 = call <vilib>:"DAQmx Clear Task.vi"("task in"=w284, "error in"=w282) -> ("error out"=→"error out 45":errorcluster)  [unwired: 13 in]
      }
      frame "5" {
        n151 = call-poly <vilib>:"DAQmx Create Virtual Channel.vi"("lines"=tag "myDAQ1/port0/line0") -> ("task out"=w359:refnum<k21>, "error out"=w357:errorcluster)  [unwired: 13 in]
        n152 = call-poly <vilib>:"DAQmx Create Virtual Channel.vi"("lines"=tag "myDAQ1/port0/line1") -> ("task out"=w335:refnum<k21>, "error out"=w333:errorcluster)  [unwired: 13 in]
        n153 = call-poly <vilib>:"DAQmx Write.vi"("task/channels in"=w359, "data"=bool[] [FALSE], "error in"=w357) -> ("task out"=w358:refnum<k21>, "error out"=w356:errorcluster)  [unwired: 10 in, 1 out]
        n154 = call-poly <vilib>:"DAQmx Write.vi"("task/channels in"=w335, "data"=bool[] [FALSE], "error in"=w333) -> ("task out"=w334:refnum<k21>, "error out"=w332:errorcluster)  [unwired: 10 in, 1 out]
        n155 = call <vilib>:"DAQmx Clear Task.vi"("task in"=w358, "error in"=w356) -> ("error out"=→"error out 50":errorcluster)  [unwired: 13 in]
        n156 = call <vilib>:"DAQmx Clear Task.vi"("task in"=w334, "error in"=w332) -> ("error out"=→"error out 54":errorcluster)  [unwired: 13 in]
        n157 = call-poly <vilib>:"DAQmx Create Virtual Channel.vi"("lines"=tag "myDAQ1/port0/line3") -> ("task out"=w329:refnum<k21>, "error out"=w327:errorcluster)  [unwired: 13 in]
        n158 = call-poly <vilib>:"DAQmx Create Virtual Channel.vi"("lines"=tag "myDAQ1/port0/line2") -> ("task out"=w353:refnum<k21>, "error out"=w351:errorcluster)  [unwired: 13 in]
        n159 = call-poly <vilib>:"DAQmx Write.vi"("task/channels in"=w329, "data"=bool[] [FALSE], "error in"=w327) -> ("task out"=w328:refnum<k21>, "error out"=w326:errorcluster)  [unwired: 10 in, 1 out]
        n160 = call-poly <vilib>:"DAQmx Write.vi"("task/channels in"=w353, "data"=bool[] [FALSE], "error in"=w351) -> ("task out"=w352:refnum<k21>, "error out"=w350:errorcluster)  [unwired: 10 in, 1 out]
        n161 = call <vilib>:"DAQmx Clear Task.vi"("task in"=w328, "error in"=w326) -> ("error out"=→"error out 55":errorcluster)  [unwired: 13 in]
        n162 = call <vilib>:"DAQmx Clear Task.vi"("task in"=w352, "error in"=w350) -> ("error out"=→"error out 51":errorcluster)  [unwired: 13 in]
        n163 = call-poly <vilib>:"DAQmx Create Virtual Channel.vi"("lines"=tag "myDAQ1/port0/line5") -> ("task out"=w323:refnum<k21>, "error out"=w321:errorcluster)  [unwired: 13 in]
        n164 = call-poly <vilib>:"DAQmx Write.vi"("task/channels in"=w323, "data"=bool[] [FALSE], "error in"=w321) -> ("task out"=w322:refnum<k21>, "error out"=w320:errorcluster)  [unwired: 10 in, 1 out]
        n165 = call-poly <vilib>:"DAQmx Create Virtual Channel.vi"("lines"=tag "myDAQ1/port0/line4") -> ("task out"=w347:refnum<k21>, "error out"=w345:errorcluster)  [unwired: 13 in]
        n166 = call <vilib>:"DAQmx Clear Task.vi"("task in"=w322, "error in"=w320) -> ("error out"=→"error out 56":errorcluster)  [unwired: 13 in]
        n167 = call-poly <vilib>:"DAQmx Write.vi"("task/channels in"=w347, "data"=bool[] [TRUE], "error in"=w345) -> ("task out"=w346:refnum<k21>, "error out"=w344:errorcluster)  [unwired: 10 in, 1 out]
        n168 = call <vilib>:"DAQmx Clear Task.vi"("task in"=w346, "error in"=w344) -> ("error out"=→"error out 52":errorcluster)  [unwired: 13 in]
        n169 = call-poly <vilib>:"DAQmx Create Virtual Channel.vi"("lines"=tag "myDAQ1/port0/line7") -> ("task out"=w317:refnum<k21>, "error out"=w315:errorcluster)  [unwired: 13 in]
        n170 = call-poly <vilib>:"DAQmx Write.vi"("task/channels in"=w317, "data"=bool[] [FALSE], "error in"=w315) -> ("task out"=w316:refnum<k21>, "error out"=w314:errorcluster)  [unwired: 10 in, 1 out]
        n171 = call-poly <vilib>:"DAQmx Create Virtual Channel.vi"("lines"=tag "myDAQ1/port0/line6") -> ("task out"=w341:refnum<k21>, "error out"=w339:errorcluster)  [unwired: 13 in]
        n172 = call <vilib>:"DAQmx Clear Task.vi"("task in"=w316, "error in"=w314) -> ("error out"=→"error out 57":errorcluster)  [unwired: 13 in]
        n173 = call-poly <vilib>:"DAQmx Write.vi"("task/channels in"=w341, "data"=bool[] [FALSE], "error in"=w339) -> ("task out"=w340:refnum<k21>, "error out"=w338:errorcluster)  [unwired: 10 in, 1 out]
        n174 = call <vilib>:"DAQmx Clear Task.vi"("task in"=w340, "error in"=w338) -> ("error out"=→"error out 53":errorcluster)  [unwired: 13 in]
      }
      frame "6" {
        n175 = call-poly <vilib>:"DAQmx Create Virtual Channel.vi"("lines"=tag "myDAQ1/port0/line0") -> ("task out"=w415:refnum<k21>, "error out"=w413:errorcluster)  [unwired: 13 in]
        n176 = call-poly <vilib>:"DAQmx Create Virtual Channel.vi"("lines"=tag "myDAQ1/port0/line1") -> ("task out"=w391:refnum<k21>, "error out"=w389:errorcluster)  [unwired: 13 in]
        n177 = call-poly <vilib>:"DAQmx Write.vi"("task/channels in"=w415, "data"=bool[] [FALSE], "error in"=w413) -> ("task out"=w414:refnum<k21>, "error out"=w412:errorcluster)  [unwired: 10 in, 1 out]
        n178 = call-poly <vilib>:"DAQmx Write.vi"("task/channels in"=w391, "data"=bool[] [FALSE], "error in"=w389) -> ("task out"=w390:refnum<k21>, "error out"=w388:errorcluster)  [unwired: 10 in, 1 out]
        n179 = call <vilib>:"DAQmx Clear Task.vi"("task in"=w414, "error in"=w412) -> ("error out"=→"error out 58":errorcluster)  [unwired: 13 in]
        n180 = call <vilib>:"DAQmx Clear Task.vi"("task in"=w390, "error in"=w388) -> ("error out"=→"error out 62":errorcluster)  [unwired: 13 in]
        n181 = call-poly <vilib>:"DAQmx Create Virtual Channel.vi"("lines"=tag "myDAQ1/port0/line3") -> ("task out"=w385:refnum<k21>, "error out"=w383:errorcluster)  [unwired: 13 in]
        n182 = call-poly <vilib>:"DAQmx Create Virtual Channel.vi"("lines"=tag "myDAQ1/port0/line2") -> ("task out"=w409:refnum<k21>, "error out"=w407:errorcluster)  [unwired: 13 in]
        n183 = call-poly <vilib>:"DAQmx Write.vi"("task/channels in"=w385, "data"=bool[] [FALSE], "error in"=w383) -> ("task out"=w384:refnum<k21>, "error out"=w382:errorcluster)  [unwired: 10 in, 1 out]
        n184 = call-poly <vilib>:"DAQmx Write.vi"("task/channels in"=w409, "data"=bool[] [FALSE], "error in"=w407) -> ("task out"=w408:refnum<k21>, "error out"=w406:errorcluster)  [unwired: 10 in, 1 out]
        n185 = call <vilib>:"DAQmx Clear Task.vi"("task in"=w384, "error in"=w382) -> ("error out"=→"error out 63":errorcluster)  [unwired: 13 in]
        n186 = call <vilib>:"DAQmx Clear Task.vi"("task in"=w408, "error in"=w406) -> ("error out"=→"error out 59":errorcluster)  [unwired: 13 in]
        n187 = call-poly <vilib>:"DAQmx Create Virtual Channel.vi"("lines"=tag "myDAQ1/port0/line5") -> ("task out"=w379:refnum<k21>, "error out"=w377:errorcluster)  [unwired: 13 in]
        n188 = call-poly <vilib>:"DAQmx Write.vi"("task/channels in"=w379, "data"=bool[] [TRUE], "error in"=w377) -> ("task out"=w378:refnum<k21>, "error out"=w376:errorcluster)  [unwired: 10 in, 1 out]
        n189 = call-poly <vilib>:"DAQmx Create Virtual Channel.vi"("lines"=tag "myDAQ1/port0/line4") -> ("task out"=w403:refnum<k21>, "error out"=w401:errorcluster)  [unwired: 13 in]
        n190 = call <vilib>:"DAQmx Clear Task.vi"("task in"=w378, "error in"=w376) -> ("error out"=→"error out 64":errorcluster)  [unwired: 13 in]
        n191 = call-poly <vilib>:"DAQmx Write.vi"("task/channels in"=w403, "data"=bool[] [FALSE], "error in"=w401) -> ("task out"=w402:refnum<k21>, "error out"=w400:errorcluster)  [unwired: 10 in, 1 out]
        n192 = call <vilib>:"DAQmx Clear Task.vi"("task in"=w402, "error in"=w400) -> ("error out"=→"error out 60":errorcluster)  [unwired: 13 in]
        n193 = call-poly <vilib>:"DAQmx Create Virtual Channel.vi"("lines"=tag "myDAQ1/port0/line7") -> ("task out"=w373:refnum<k21>, "error out"=w371:errorcluster)  [unwired: 13 in]
        n194 = call-poly <vilib>:"DAQmx Write.vi"("task/channels in"=w373, "data"=bool[] [FALSE], "error in"=w371) -> ("task out"=w372:refnum<k21>, "error out"=w370:errorcluster)  [unwired: 10 in, 1 out]
        n195 = call-poly <vilib>:"DAQmx Create Virtual Channel.vi"("lines"=tag "myDAQ1/port0/line6") -> ("task out"=w397:refnum<k21>, "error out"=w395:errorcluster)  [unwired: 13 in]
        n196 = call <vilib>:"DAQmx Clear Task.vi"("task in"=w372, "error in"=w370) -> ("error out"=→"error out 65":errorcluster)  [unwired: 13 in]
        n197 = call-poly <vilib>:"DAQmx Write.vi"("task/channels in"=w397, "data"=bool[] [FALSE], "error in"=w395) -> ("task out"=w396:refnum<k21>, "error out"=w394:errorcluster)  [unwired: 10 in, 1 out]
        n198 = call <vilib>:"DAQmx Clear Task.vi"("task in"=w396, "error in"=w394) -> ("error out"=→"error out 61":errorcluster)  [unwired: 13 in]
      }
      frame "7" {
        n199 = call-poly <vilib>:"DAQmx Create Virtual Channel.vi"("lines"=tag "myDAQ1/port0/line0") -> ("task out"=w471:refnum<k21>, "error out"=w469:errorcluster)  [unwired: 13 in]
        n200 = call-poly <vilib>:"DAQmx Create Virtual Channel.vi"("lines"=tag "myDAQ1/port0/line1") -> ("task out"=w447:refnum<k21>, "error out"=w445:errorcluster)  [unwired: 13 in]
        n201 = call-poly <vilib>:"DAQmx Write.vi"("task/channels in"=w471, "data"=bool[] [FALSE], "error in"=w469) -> ("task out"=w470:refnum<k21>, "error out"=w468:errorcluster)  [unwired: 10 in, 1 out]
        n202 = call-poly <vilib>:"DAQmx Write.vi"("task/channels in"=w447, "data"=bool[] [FALSE], "error in"=w445) -> ("task out"=w446:refnum<k21>, "error out"=w444:errorcluster)  [unwired: 10 in, 1 out]
        n203 = call <vilib>:"DAQmx Clear Task.vi"("task in"=w470, "error in"=w468) -> ("error out"=→"error out 66":errorcluster)  [unwired: 13 in]
        n204 = call <vilib>:"DAQmx Clear Task.vi"("task in"=w446, "error in"=w444) -> ("error out"=→"error out 70":errorcluster)  [unwired: 13 in]
        n205 = call-poly <vilib>:"DAQmx Create Virtual Channel.vi"("lines"=tag "myDAQ1/port0/line3") -> ("task out"=w441:refnum<k21>, "error out"=w439:errorcluster)  [unwired: 13 in]
        n206 = call-poly <vilib>:"DAQmx Create Virtual Channel.vi"("lines"=tag "myDAQ1/port0/line2") -> ("task out"=w465:refnum<k21>, "error out"=w463:errorcluster)  [unwired: 13 in]
        n207 = call-poly <vilib>:"DAQmx Write.vi"("task/channels in"=w441, "data"=bool[] [FALSE], "error in"=w439) -> ("task out"=w440:refnum<k21>, "error out"=w438:errorcluster)  [unwired: 10 in, 1 out]
        n208 = call-poly <vilib>:"DAQmx Write.vi"("task/channels in"=w465, "data"=bool[] [FALSE], "error in"=w463) -> ("task out"=w464:refnum<k21>, "error out"=w462:errorcluster)  [unwired: 10 in, 1 out]
        n209 = call <vilib>:"DAQmx Clear Task.vi"("task in"=w440, "error in"=w438) -> ("error out"=→"error out 71":errorcluster)  [unwired: 13 in]
        n210 = call <vilib>:"DAQmx Clear Task.vi"("task in"=w464, "error in"=w462) -> ("error out"=→"error out 67":errorcluster)  [unwired: 13 in]
        n211 = call-poly <vilib>:"DAQmx Create Virtual Channel.vi"("lines"=tag "myDAQ1/port0/line5") -> ("task out"=w435:refnum<k21>, "error out"=w433:errorcluster)  [unwired: 13 in]
        n212 = call-poly <vilib>:"DAQmx Write.vi"("task/channels in"=w435, "data"=bool[] [FALSE], "error in"=w433) -> ("task out"=w434:refnum<k21>, "error out"=w432:errorcluster)  [unwired: 10 in, 1 out]
        n213 = call-poly <vilib>:"DAQmx Create Virtual Channel.vi"("lines"=tag "myDAQ1/port0/line4") -> ("task out"=w459:refnum<k21>, "error out"=w457:errorcluster)  [unwired: 13 in]
        n214 = call <vilib>:"DAQmx Clear Task.vi"("task in"=w434, "error in"=w432) -> ("error out"=→"error out 72":errorcluster)  [unwired: 13 in]
        n215 = call-poly <vilib>:"DAQmx Write.vi"("task/channels in"=w459, "data"=bool[] [FALSE], "error in"=w457) -> ("task out"=w458:refnum<k21>, "error out"=w456:errorcluster)  [unwired: 10 in, 1 out]
        n216 = call <vilib>:"DAQmx Clear Task.vi"("task in"=w458, "error in"=w456) -> ("error out"=→"error out 68":errorcluster)  [unwired: 13 in]
        n217 = call-poly <vilib>:"DAQmx Create Virtual Channel.vi"("lines"=tag "myDAQ1/port0/line7") -> ("task out"=w429:refnum<k21>, "error out"=w427:errorcluster)  [unwired: 13 in]
        n218 = call-poly <vilib>:"DAQmx Write.vi"("task/channels in"=w429, "data"=bool[] [FALSE], "error in"=w427) -> ("task out"=w428:refnum<k21>, "error out"=w426:errorcluster)  [unwired: 10 in, 1 out]
        n219 = call-poly <vilib>:"DAQmx Create Virtual Channel.vi"("lines"=tag "myDAQ1/port0/line6") -> ("task out"=w453:refnum<k21>, "error out"=w451:errorcluster)  [unwired: 13 in]
        n220 = call <vilib>:"DAQmx Clear Task.vi"("task in"=w428, "error in"=w426) -> ("error out"=→"error out 73":errorcluster)  [unwired: 13 in]
        n221 = call-poly <vilib>:"DAQmx Write.vi"("task/channels in"=w453, "data"=bool[] [TRUE], "error in"=w451) -> ("task out"=w452:refnum<k21>, "error out"=w450:errorcluster)  [unwired: 10 in, 1 out]
        n222 = call <vilib>:"DAQmx Clear Task.vi"("task in"=w452, "error in"=w450) -> ("error out"=→"error out 69":errorcluster)  [unwired: 13 in]
      }
      frame "8" {
        n223 = call-poly <vilib>:"DAQmx Create Virtual Channel.vi"("lines"=tag "myDAQ1/port0/line0") -> ("task out"=w527:refnum<k21>, "error out"=w525:errorcluster)  [unwired: 13 in]
        n224 = call-poly <vilib>:"DAQmx Create Virtual Channel.vi"("lines"=tag "myDAQ1/port0/line1") -> ("task out"=w503:refnum<k21>, "error out"=w501:errorcluster)  [unwired: 13 in]
        n225 = call-poly <vilib>:"DAQmx Write.vi"("task/channels in"=w527, "data"=bool[] [FALSE], "error in"=w525) -> ("task out"=w526:refnum<k21>, "error out"=w524:errorcluster)  [unwired: 10 in, 1 out]
        n226 = call-poly <vilib>:"DAQmx Write.vi"("task/channels in"=w503, "data"=bool[] [FALSE], "error in"=w501) -> ("task out"=w502:refnum<k21>, "error out"=w500:errorcluster)  [unwired: 10 in, 1 out]
        n227 = call <vilib>:"DAQmx Clear Task.vi"("task in"=w526, "error in"=w524) -> ("error out"=→"error out 74":errorcluster)  [unwired: 13 in]
        n228 = call <vilib>:"DAQmx Clear Task.vi"("task in"=w502, "error in"=w500) -> ("error out"=→"error out 78":errorcluster)  [unwired: 13 in]
        n229 = call-poly <vilib>:"DAQmx Create Virtual Channel.vi"("lines"=tag "myDAQ1/port0/line3") -> ("task out"=w497:refnum<k21>, "error out"=w495:errorcluster)  [unwired: 13 in]
        n230 = call-poly <vilib>:"DAQmx Create Virtual Channel.vi"("lines"=tag "myDAQ1/port0/line2") -> ("task out"=w521:refnum<k21>, "error out"=w519:errorcluster)  [unwired: 13 in]
        n231 = call-poly <vilib>:"DAQmx Write.vi"("task/channels in"=w497, "data"=bool[] [FALSE], "error in"=w495) -> ("task out"=w496:refnum<k21>, "error out"=w494:errorcluster)  [unwired: 10 in, 1 out]
        n232 = call-poly <vilib>:"DAQmx Write.vi"("task/channels in"=w521, "data"=bool[] [FALSE], "error in"=w519) -> ("task out"=w520:refnum<k21>, "error out"=w518:errorcluster)  [unwired: 10 in, 1 out]
        n233 = call <vilib>:"DAQmx Clear Task.vi"("task in"=w496, "error in"=w494) -> ("error out"=→"error out 79":errorcluster)  [unwired: 13 in]
        n234 = call <vilib>:"DAQmx Clear Task.vi"("task in"=w520, "error in"=w518) -> ("error out"=→"error out 75":errorcluster)  [unwired: 13 in]
        n235 = call-poly <vilib>:"DAQmx Create Virtual Channel.vi"("lines"=tag "myDAQ1/port0/line5") -> ("task out"=w491:refnum<k21>, "error out"=w489:errorcluster)  [unwired: 13 in]
        n236 = call-poly <vilib>:"DAQmx Write.vi"("task/channels in"=w491, "data"=bool[] [FALSE], "error in"=w489) -> ("task out"=w490:refnum<k21>, "error out"=w488:errorcluster)  [unwired: 10 in, 1 out]
        n237 = call-poly <vilib>:"DAQmx Create Virtual Channel.vi"("lines"=tag "myDAQ1/port0/line4") -> ("task out"=w515:refnum<k21>, "error out"=w513:errorcluster)  [unwired: 13 in]
        n238 = call <vilib>:"DAQmx Clear Task.vi"("task in"=w490, "error in"=w488) -> ("error out"=→"error out 80":errorcluster)  [unwired: 13 in]
        n239 = call-poly <vilib>:"DAQmx Write.vi"("task/channels in"=w515, "data"=bool[] [FALSE], "error in"=w513) -> ("task out"=w514:refnum<k21>, "error out"=w512:errorcluster)  [unwired: 10 in, 1 out]
        n240 = call <vilib>:"DAQmx Clear Task.vi"("task in"=w514, "error in"=w512) -> ("error out"=→"error out 76":errorcluster)  [unwired: 13 in]
        n241 = call-poly <vilib>:"DAQmx Create Virtual Channel.vi"("lines"=tag "myDAQ1/port0/line7") -> ("task out"=w485:refnum<k21>, "error out"=w483:errorcluster)  [unwired: 13 in]
        n242 = call-poly <vilib>:"DAQmx Write.vi"("task/channels in"=w485, "data"=bool[] [TRUE], "error in"=w483) -> ("task out"=w484:refnum<k21>, "error out"=w482:errorcluster)  [unwired: 10 in, 1 out]
        n243 = call-poly <vilib>:"DAQmx Create Virtual Channel.vi"("lines"=tag "myDAQ1/port0/line6") -> ("task out"=w509:refnum<k21>, "error out"=w507:errorcluster)  [unwired: 13 in]
        n244 = call <vilib>:"DAQmx Clear Task.vi"("task in"=w484, "error in"=w482) -> ("error out"=→"error out 81":errorcluster)  [unwired: 13 in]
        n245 = call-poly <vilib>:"DAQmx Write.vi"("task/channels in"=w509, "data"=bool[] [FALSE], "error in"=w507) -> ("task out"=w508:refnum<k21>, "error out"=w506:errorcluster)  [unwired: 10 in, 1 out]
        n246 = call <vilib>:"DAQmx Clear Task.vi"("task in"=w508, "error in"=w506) -> ("error out"=→"error out 77":errorcluster)  [unwired: 13 in]
      }
      frame "9" {
        n247 = call-poly <vilib>:"DAQmx Create Virtual Channel.vi"("lines"=tag "myDAQ1/port0/line0") -> ("task out"=w583:refnum<k21>, "error out"=w581:errorcluster)  [unwired: 13 in]
        n248 = call-poly <vilib>:"DAQmx Create Virtual Channel.vi"("lines"=tag "myDAQ1/port0/line1") -> ("task out"=w559:refnum<k21>, "error out"=w557:errorcluster)  [unwired: 13 in]
        n249 = call-poly <vilib>:"DAQmx Write.vi"("task/channels in"=w583, "data"=bool[] [FALSE], "error in"=w581) -> ("task out"=w582:refnum<k21>, "error out"=w580:errorcluster)  [unwired: 10 in, 1 out]
        n250 = call-poly <vilib>:"DAQmx Write.vi"("task/channels in"=w559, "data"=bool[] [TRUE], "error in"=w557) -> ("task out"=w558:refnum<k21>, "error out"=w556:errorcluster)  [unwired: 10 in, 1 out]
        n251 = call <vilib>:"DAQmx Clear Task.vi"("task in"=w582, "error in"=w580) -> ("error out"=→"error out 90":errorcluster)  [unwired: 13 in]
        n252 = call <vilib>:"DAQmx Clear Task.vi"("task in"=w558, "error in"=w556) -> ("error out"=→"error out 94":errorcluster)  [unwired: 13 in]
        n253 = call-poly <vilib>:"DAQmx Create Virtual Channel.vi"("lines"=tag "myDAQ1/port0/line3") -> ("task out"=w553:refnum<k21>, "error out"=w551:errorcluster)  [unwired: 13 in]
        n254 = call-poly <vilib>:"DAQmx Create Virtual Channel.vi"("lines"=tag "myDAQ1/port0/line2") -> ("task out"=w577:refnum<k21>, "error out"=w575:errorcluster)  [unwired: 13 in]
        n255 = call-poly <vilib>:"DAQmx Write.vi"("task/channels in"=w553, "data"=bool[] [TRUE], "error in"=w551) -> ("task out"=w552:refnum<k21>, "error out"=w550:errorcluster)  [unwired: 10 in, 1 out]
        n256 = call-poly <vilib>:"DAQmx Write.vi"("task/channels in"=w577, "data"=bool[] [FALSE], "error in"=w575) -> ("task out"=w576:refnum<k21>, "error out"=w574:errorcluster)  [unwired: 10 in, 1 out]
        n257 = call <vilib>:"DAQmx Clear Task.vi"("task in"=w552, "error in"=w550) -> ("error out"=→"error out 95":errorcluster)  [unwired: 13 in]
        n258 = call <vilib>:"DAQmx Clear Task.vi"("task in"=w576, "error in"=w574) -> ("error out"=→"error out 91":errorcluster)  [unwired: 13 in]
        n259 = call-poly <vilib>:"DAQmx Create Virtual Channel.vi"("lines"=tag "myDAQ1/port0/line5") -> ("task out"=w547:refnum<k21>, "error out"=w545:errorcluster)  [unwired: 13 in]
        n260 = call-poly <vilib>:"DAQmx Write.vi"("task/channels in"=w547, "data"=bool[] [TRUE], "error in"=w545) -> ("task out"=w546:refnum<k21>, "error out"=w544:errorcluster)  [unwired: 10 in, 1 out]
        n261 = call-poly <vilib>:"DAQmx Create Virtual Channel.vi"("lines"=tag "myDAQ1/port0/line4") -> ("task out"=w571:refnum<k21>, "error out"=w569:errorcluster)  [unwired: 13 in]
        n262 = call <vilib>:"DAQmx Clear Task.vi"("task in"=w546, "error in"=w544) -> ("error out"=→"error out 96":errorcluster)  [unwired: 13 in]
        n263 = call-poly <vilib>:"DAQmx Write.vi"("task/channels in"=w571, "data"=bool[] [FALSE], "error in"=w569) -> ("task out"=w570:refnum<k21>, "error out"=w568:errorcluster)  [unwired: 10 in, 1 out]
        n264 = call <vilib>:"DAQmx Clear Task.vi"("task in"=w570, "error in"=w568) -> ("error out"=→"error out 92":errorcluster)  [unwired: 13 in]
        n265 = call-poly <vilib>:"DAQmx Create Virtual Channel.vi"("lines"=tag "myDAQ1/port0/line7") -> ("task out"=w541:refnum<k21>, "error out"=w539:errorcluster)  [unwired: 13 in]
        n266 = call-poly <vilib>:"DAQmx Write.vi"("task/channels in"=w541, "data"=bool[] [TRUE], "error in"=w539) -> ("task out"=w540:refnum<k21>, "error out"=w538:errorcluster)  [unwired: 10 in, 1 out]
        n267 = call-poly <vilib>:"DAQmx Create Virtual Channel.vi"("lines"=tag "myDAQ1/port0/line6") -> ("task out"=w565:refnum<k21>, "error out"=w563:errorcluster)  [unwired: 13 in]
        n268 = call <vilib>:"DAQmx Clear Task.vi"("task in"=w540, "error in"=w538) -> ("error out"=→"error out 97":errorcluster)  [unwired: 13 in]
        n269 = call-poly <vilib>:"DAQmx Write.vi"("task/channels in"=w565, "data"=bool[] [FALSE], "error in"=w563) -> ("task out"=w564:refnum<k21>, "error out"=w562:errorcluster)  [unwired: 10 in, 1 out]
        n270 = call <vilib>:"DAQmx Clear Task.vi"("task in"=w564, "error in"=w562) -> ("error out"=→"error out 93":errorcluster)  [unwired: 13 in]
      }
    }
    n271 = Add(x=1, y=w11) -> (x+y=w10:dbl)
  }
